vi "Main.vi"() -> ()   [LabVIEW 2017]
uses:
  type defs/action buttons.ctl
  type defs/mode buttons.ctl
  <vilib>/vision/Pattern Matching.llb/IMAQ GM Match Report.ctl
  type defs/data.ctl
  <vilib>/vision/Image Controls.llb/IMAQ Image.ctl
  type defs/states.ctl
  <vilib>/myRIO/Instrument Drivers/Onboard IO/PWM/typedefs/PWM Reference.ctl
  <vilib>/myRIO/Common/Instrument Driver Framework/Utilities/typedefs/myRIO Generic Hardware Reference.ctl
  <vilib>/myRIO/Common/Instrument Driver Framework/Utilities/typedefs/Hardware Version Enum.ctl
  <vilib>/myRIO/Common/Instrument Driver Framework/Utilities/typedefs/myRIO v1.0 Reference.ctl
  <vilib>/myRIO/Common/Instrument Driver Framework/Utilities/typedefs/Generic FPGA Reference.ctl
  <vilib>/myRIO/Common/Instrument Driver Framework/myRIO v1.0/PWM/typedefs/PWM Channels Enum.ctl
  <vilib>/myRIO/Instrument Drivers/Onboard IO/PWM/typedefs/PWM Configuration.ctl
  <vilib>/userdefined/High Color/nirio_resource_hc.ctl
  <vilib>/myRIO/Instrument Drivers/Onboard IO/DIO/typedefs/DIO Reference.ctl
  <vilib>/myRIO/Common/Instrument Driver Framework/myRIO v1.0/DIO/typedefs/DIO Channels List.ctl
  <vilib>/myRIO/Common/Instrument Driver Framework/myRIO v1.0/DIO/typedefs/DIO Channels Enum.ctl
  type defs/task.ctl
  <vilib>/myRIO/Common/Instrument Driver Framework/Utilities/vis/Is FPGA Ref Available.vi
  <vilib>/myRIO/Common/Instrument Driver Framework/myRIO v1.0/PWM/vis/myRIO v1.1 Open PWM.vi
  <vilib>/myRIO/Instrument Drivers/Onboard IO/PWM/vis/Set Duty Cycle and Frequency.vi
  <vilib>/myRIO/Common/Instrument Driver Framework/myRIO v1.0/DIO/vis/myRIO v1.1 Open DIO.vi
  <vilib>/myRIO/Instrument Drivers/Onboard IO/DIO/vis/Write.vi
  <vilib>/myRIO/Instrument Drivers/Onboard IO/DIO/vis/Read.vi
  <vilib>/myRIO/Common/Instrument Driver Framework/Utilities/vis/Validate Channels.vi
  <vilib>/myRIO/Common/Instrument Driver Framework/myRIO v1.0/PWM/vis/myRIO v1.0 Reserve PWM.vi
  <vilib>/myRIO/Common/Instrument Driver Framework/myRIO v1.0/DIO/vis/myRIO v1.0 Reserve DIO.vi
  <vilib>/myRIO/Common/Instrument Driver Framework/myRIO v1.0/UART/vis/myRIO v1.0 Close UART.vi
  <vilib>/myRIO/Common/Instrument Driver Framework/myRIO v1.0/PWM/vis/myRIO v1.0 Build MUX Configuration PWM.vi
  <vilib>/myRIO/Common/Instrument Driver Framework/myRIO v1.0/Resource Manager/vis/myRIO v1.0 Reserve Channel List.vi
  <vilib>/myRIO/Common/Instrument Driver Framework/myRIO v1.0/DIO/vis/myRIO v1.0 Build MUX Configuration DIO.vi
  <vilib>/myRIO/Common/Instrument Driver Framework/myRIO v1.0/Resource Manager/vis/myRIO v1.0 Create Configuration List.vi
  <vilib>/myRIO/Common/Instrument Driver Framework/myRIO v1.0/Resource Manager/vis/myRIO v1.0 Reserve Channel.vi
  <vilib>/myRIO/Common/Instrument Driver Framework/myRIO v1.0/Resource Manager/vis/myRIO v1.0 Unreserve Channel.vi
  <vilib>/myRIO/Common/Instrument Driver Framework/myRIO v1.0/Resource Manager/vis/myRIO v1.0 Build Mutex Name.vi
  <vilib>/Utility/VariantDataType/GetNumericInfo.vi
  <vilib>/Utility/error.llb/Error Cluster From Error Code.vi
  <vilib>/myRIO/Common/Instrument Driver Framework/myRIO v1.0/myRIO v1.1 Open.vi
  <vilib>/myRIO/Common/Instrument Driver Framework/Utilities/vis/IO Manager.vi
  <vilib>/myRIO/Common/Instrument Driver Framework/Utilities/vis/Configuration Manager.vi
  <vilib>/myRIO/Common/Instrument Driver Framework/myRIO v1.0/Resource Manager/vis/myRIO v1.0 Configure IO.vi
  <vilib>/myRIO/Common/Instrument Driver Framework/myRIO v1.0/myRIO v1.0 Close.vi
  <vilib>/myRIO/Common/Instrument Driver Framework/myRIO v1.0/PWM/vis/myRIO v1.0 Write PWM.vi
  <vilib>/myRIO/Common/Instrument Driver Framework/myRIO v1.0/DIO/vis/myRIO v1.0 Write DIO.vi
  <vilib>/myRIO/Common/Instrument Driver Framework/myRIO v1.0/DIO/vis/myRIO v1.0 Read DIO.vi
  <vilib>/myRIO/Common/Instrument Driver Framework/Utilities/vis/FPGA Ref Manager.vi
  <vilib>/myRIO/Common/Instrument Driver Framework/myRIO v1.0/myRIO v1.0 Reset FPGA.vi
  <vilib>/myRIO/Common/Instrument Driver Framework/myRIO v1.0/IRQ/vis/myRIO v1.0 IRQ Info FGV.vi
  <vilib>/myRIO/Common/Instrument Driver Framework/myRIO v1.0/IRQ/vis/myRIO v1.0 Timer IRQ Info FGV.vi
  <vilib>/myRIO/Common/Instrument Driver Framework/myRIO v1.0/IRQ/vis/myRIO v1.0 ISR Agent.vi
  <vilib>/myRIO/Express VI/Onboard IO/PWM/PWM Express VI.xnode
  <vilib>/myRIO/Instrument Drivers/Onboard IO/PWM/vis/myRIO PWM Open.xnode
  <vilib>/myRIO/Express VI/Onboard IO/DO/DO Express VI.xnode
  <vilib>/myRIO/Instrument Drivers/Onboard IO/DIO/vis/myRIO DIO Open.xnode
  <vilib>/myRIO/Express VI/Onboard Devices/LED/LED Express VI.xnode
  <vilib>/myRIO/Express VI/Onboard Devices/Button/Button Express VI.xnode
  <vilib>/vision/NI_Vision_Development_Module.lvlib
  <vilib>/myRIO/Instrument Drivers/Onboard IO/DIO/DIO.lvlib
  <vilib>/myRIO/Instrument Drivers/Onboard IO/PWM/PWM.lvlib
  <vilib>/myRIO/Instrument Drivers/Utilities/Utilities.lvlib
panel:
  out "___Test___":i32[](array[numeric])
  out "data":T1={"Shape - t, Color - f"=FALSE, "qsm"={"Webcam image ref"=refnum, "Analyzed image ref"=refnum, "Stop webcam"=FALSE}, " image ref"=refnum, "number img"=0, "ROI Descriptor (Image Mask 1)"={"Global Rectangle"=[109, 72, 345, 284], "Contours"=[{"ID"=enum."External", "Type"=3, "Coordinates"=[109, 72, 345, 284]}]}, "Pattern class"=0, "Color class"=0, "ROI Descriptor COLOR Mask"={"Global Rectangle"=[109, 72, 345, 284], "Contours"=[{"ID"=enum."External", "Type"=3, "Coordinates"=[109, 72, 345, 284]}]}, "___Test___"=[]} {"ROI Descriptor COLOR Mask"."Contours"."Type" items=["No Selection", "Point", "Line", "Rectangle", "Oval", "Polygon", "Freehand Region", "Annulus", "Unused2", "Unused3", "Broken Line", "Freehand Line", "Rotated Rectangle"]; "ROI Descriptor (Image Mask 1)"."Contours"."Type" items=["No Selection", "Point", "Line", "Rectangle", "Oval", "Polygon", "Freehand Region", "Annulus", "Unused2", "Unused3", "Broken Line", "Freehand Line", "Rotated Rectangle"]}
  in  "ROI Descriptor COLOR Mask":T3={"Global Rectangle"=[109, 72, 345, 284], "Contours"=[{"ID"=enum."External", "Type"=3, "Coordinates"=[109, 72, 345, 284]}]} {"Contours"."Type" items=["No Selection", "Point", "Line", "Rectangle", "Oval", "Polygon", "Freehand Region", "Annulus", "Unused2", "Unused3", "Broken Line", "Freehand Line", "Rotated Rectangle"]}
  in  "Ball index":i32
  out "y0 (circle)":i32
  out "x0 (circle)":i32
  out "x1 (circle)":i32
  out "y1 (circle)":i32
  in  "divider (circle)":sgl=1.0
  out "CircleRadius":dbl
  in  "Look at ball":bool
  in  "x = y?":bool
  in  "y":sgl=1.0
  out "Scale":sgl
  out "error out":errorcluster
  in  "Tab Control":enum32{"Motors", "Shape/Color", "Pattern"}(tab)
  in  "Left+":bool
  in  "Left-":bool
  in  "Right+":bool
  in  "Right-":bool
  in  "M+":bool
  in  "M-":bool
  in  "G+":bool
  in  "G-":bool
  in  "M_PWM":dbl=0.5
  in  "L_PWM":dbl=0.5
  in  "R_PWM":dbl=0.5
  in  "M+ (onGrab)":bool
  out "Circles Calibrated (Shape Detection 1)":T4(array[cluster]) {"Position"."Y" format="%.2f"; "Position"."X" format="%.2f"}
  out "Number of Matches (Shape Detection 1)":i32
  out "Color":i32
  in  "Circle Descriptor (Shape Detection 1)":cluster{"Min Radius":dbl, "Max Radius":dbl}={"Min Radius"=16.0, "Max Radius"=500.0}
  in  "Align X - t, Y - f":bool
  in  "grab time (ms)":u32
  out "Class (Particle Classification 1)":string
  out "y0":i32
  out "x0":i32
  out "x1":i32
  out "y1":i32
  out "Number of Matches (Geometric Matching 1)":i32
  out "Calibrated Matches (Geometric Matching 1)":T5[](array[typedef]) {"Correlation Score" format="%.2f"; "Target Template Curve Score" format="%.2f"; "Template Target Curve Score" format="%.2f"; "Bounding Box"."y" format="%.2f"; "Bounding Box"."x" format="%.2f"; "Position"."y" format="%.2f"; "Position"."x" format="%.2f"; "Score" format="%.2f"; "Scale" format="%.2f"; "Angle" format="%.2f"; "Occlusion %" format="%.2f"}
  out "curY":sgl
  out "curX":sgl
  out "Y is in range":bool
  out "X is in range":bool
  in  "defY":dbl=170.0
  in  "Range":dbl=40.0
  in  "defX":dbl=150.0
  in  "mode buttons":T6
  out "image display":T2(plugin-control)
  in  "action buttons":T7
  in  "Stop":bool
  # "Machine\nVision\nApp"
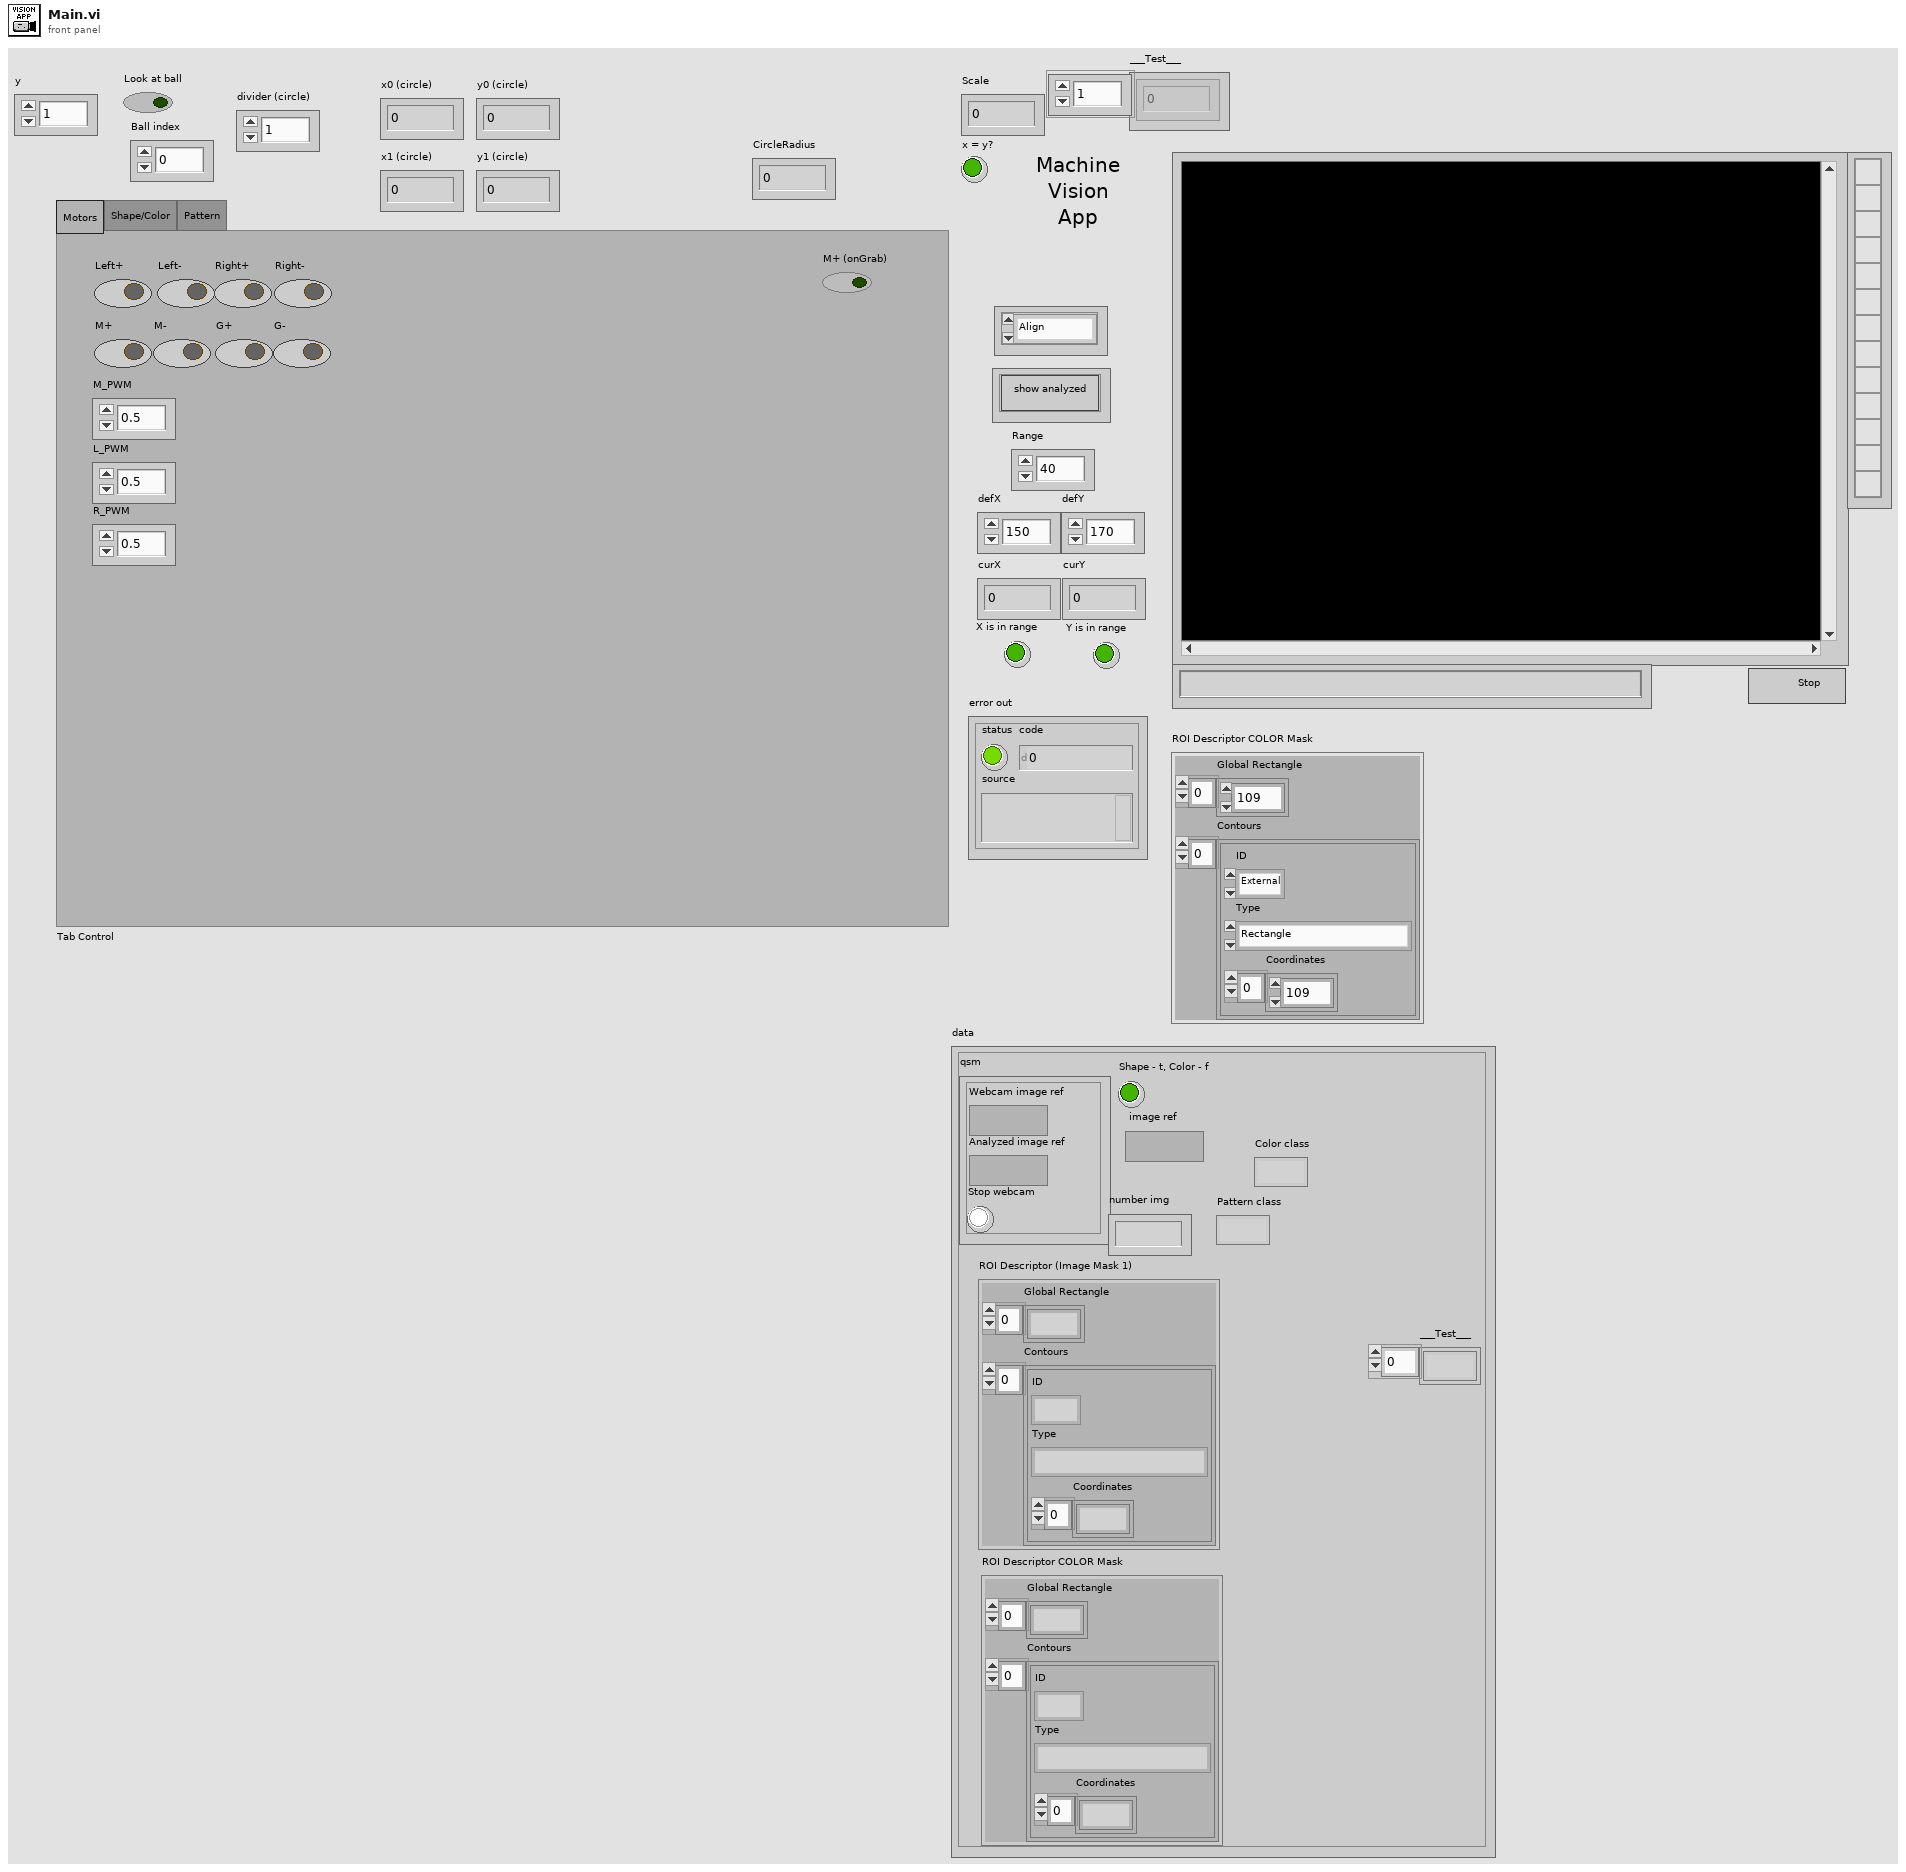
[diagram p1: front panel]
types:
  T1 = typedef "data.ctl" = cluster{"Shape - t, Color - f":bool, "qsm":cluster{"Webcam image ref":T2, "Analyzed image ref":T2, "Stop webcam":bool}, " image ref":T2, "number img":i32, "ROI Descriptor (Image Mask 1)":cluster{"Global Rectangle":i32[], "Contours":cluster{"ID":enum32{"External", "Internal"}, "Type":u32, "Coordinates":i32[]}[]}, "Pattern class":i32, "Color class":i32, "ROI Descriptor COLOR Mask":cluster{"Global Rectangle":i32[], "Contours":cluster{"ID":enum32{"External", "Internal"}, "Type":u32, "Coordinates":i32[]}[]}, "___Test___":i32[]}
  T2 = typedef "IMAQ Image.ctl" = refnum<image>
  T3 = cluster{"Global Rectangle":i32[], "Contours":cluster{"ID":enum32{"External", "Internal"}, "Type":u32, "Coordinates":i32[]}[]}
  T4 = cluster{"Position":cluster{"X":sgl, "Y":sgl}, "Radius":dbl, "Score":dbl}[]
  T5 = typedef "IMAQ GM Match Report.ctl" = cluster{"Position":cluster{"x":sgl, "y":sgl}, "Angle":sgl, "Scale":sgl, "Score":sgl, "Bounding Box":cluster{"x":sgl, "y":sgl}[], "Contrast Reversed":bool, "Occlusion %":sgl, "Template Target Curve Score":sgl, "Target Template Curve Score":sgl, "Correlation Score":sgl}
  T6 = typedef "mode buttons.ctl" = cluster{"show analyzed":bool}
  T7 = typedef "action buttons.ctl" = cluster{"Shape - t, Color - f":enum16{"Align", "Pattern", "Ball", "Other", "Clear", "Joystick control"}}
  T8 = typedef "states.ctl" = enum16{"(qsm) schedule", "(qsm) initialize", "(qsm) release", "(qsm) clean up", "(qsm) shutdown", "(myRIO) initialize", "(myRIO) clean up", "(myRIO) update ports", "(image) get", "(image) analyze", "(image) show", "(ball) Shape detection", "(ball) Calc ball indx", "(ball) Calculate ROI", "X align", "Wait", "Grab", "(pattern) Find Square", "(pattern) Calculate ROI", "(pattern) Analyze pattern", "(joystick) Joystick control", "Wait for button"}
  T9 = typedef "DIO.lvlib/DIO Reference.ctl" = cluster{"myRIO Reference":T10, "DIO Channels List":T14}
  T10 = typedef "myRIO Generic Hardware Reference.ctl" = cluster{"myRIO Model":T11, "myRIO Hardware Reference":T12}
  T11 = typedef "Hardware Version Enum.ctl" = enum16{"Unknown", "myRIO-1900", "myRIO-1950", "roboRIO", "NI ELVIS RIO CM"}
  T12 = typedef "myRIO v1.0 Reference.ctl" = cluster{"Generic FPGA Reference":T13, "Allow multiple opens":bool}
  T13 = typedef "Generic FPGA Reference.ctl" = refnum<k20>
  T14 = typedef "DIO Channels List.ctl" = T15[]
  T15 = typedef "DIO Channels Enum.ctl" = enum16{"Not Connected", "C/DIO0", "C/DIO1", "C/DIO2", "C/DIO3", "C/DIO4", "C/DIO5", "C/DIO6", "C/DIO7", "A/DIO0", "A/DIO1", "A/DIO2", "A/DIO3", "A/DIO4", "A/DIO5", "A/DIO6", "A/DIO7", "A/DIO8", "A/DIO9", "A/DIO10", "A/DIO11", "A/DIO12", "A/DIO13", "A/DIO14", "A/DIO15", "B/DIO0", "B/DIO1", "B/DIO2", "B/DIO3", "B/DIO4", "B/DIO5", "B/DIO6", "B/DIO7", "B/DIO8", "B/DIO9", "B/DIO10", "B/DIO11", "B/DIO12", "B/DIO13", "B/DIO14", "B/DIO15", "LED0", "LED1", "LED2", "LED3", "Button0", "DIO/DIO0", "DIO/DIO1", "DIO/DIO2", "DIO/DIO3", "DIO/DIO4", "DIO/DIO5", "DIO/DIO6", "DIO/DIO7", "DIO/DIO8", "DIO/DIO9", "SPI/CS0", "SPI/CS1", "SPI/CS2", "SPI/CS3", "LED RADIO (Green)", "LED RADIO (Red)", "LED COMM (Green)", "LED COMM (Red)", "LED MODE (Green)", "LED MODE (Red)"}
  T16 = typedef "nirio_resource_hc.ctl" = tag
  T17 = typedef "PWM.lvlib/PWM Reference.ctl" = cluster{"myRIO Reference":T10, "PWM Channels Enum":T18, "PWM Configuration":T19}
  T18 = typedef "PWM Channels Enum.ctl" = enum16{"Not Connected", "C/PWM0", "C/PWM1", "A/PWM0", "A/PWM1", "A/PWM2", "B/PWM0", "B/PWM1", "B/PWM2", "PWM/PWM0", "PWM/PWM1", "PWM/PWM2", "PWM/PWM3", "PWM/PWM4", "PWM/PWM5", "PWM/PWM6", "PWM/PWM7", "PWM/PWM8", "PWM/PWM9"}
  T19 = typedef "PWM.lvlib/PWM Configuration.ctl" = cluster{"Frequency":dbl, "Duty Cycle":dbl}
  T20 = enum16{"Align", "Pattern", "Ball", "Other", "Clear", "Joystick control"}
  T21 = typedef "task.ctl" = T8[]
  T22 = typedef "Image Type" = u32
  T23 = cluster{"Position":cluster{"X":sgl, "Y":sgl}, "Radius":dbl, "Score":dbl}
  T24 = cluster{"ID":enum32{"External", "Internal"}, "Type":u32, "Coordinates":i32[]}[]
  T25 = cluster{"ID":enum32{"External", "Internal"}, "Type":u32, "Coordinates":i32[]}
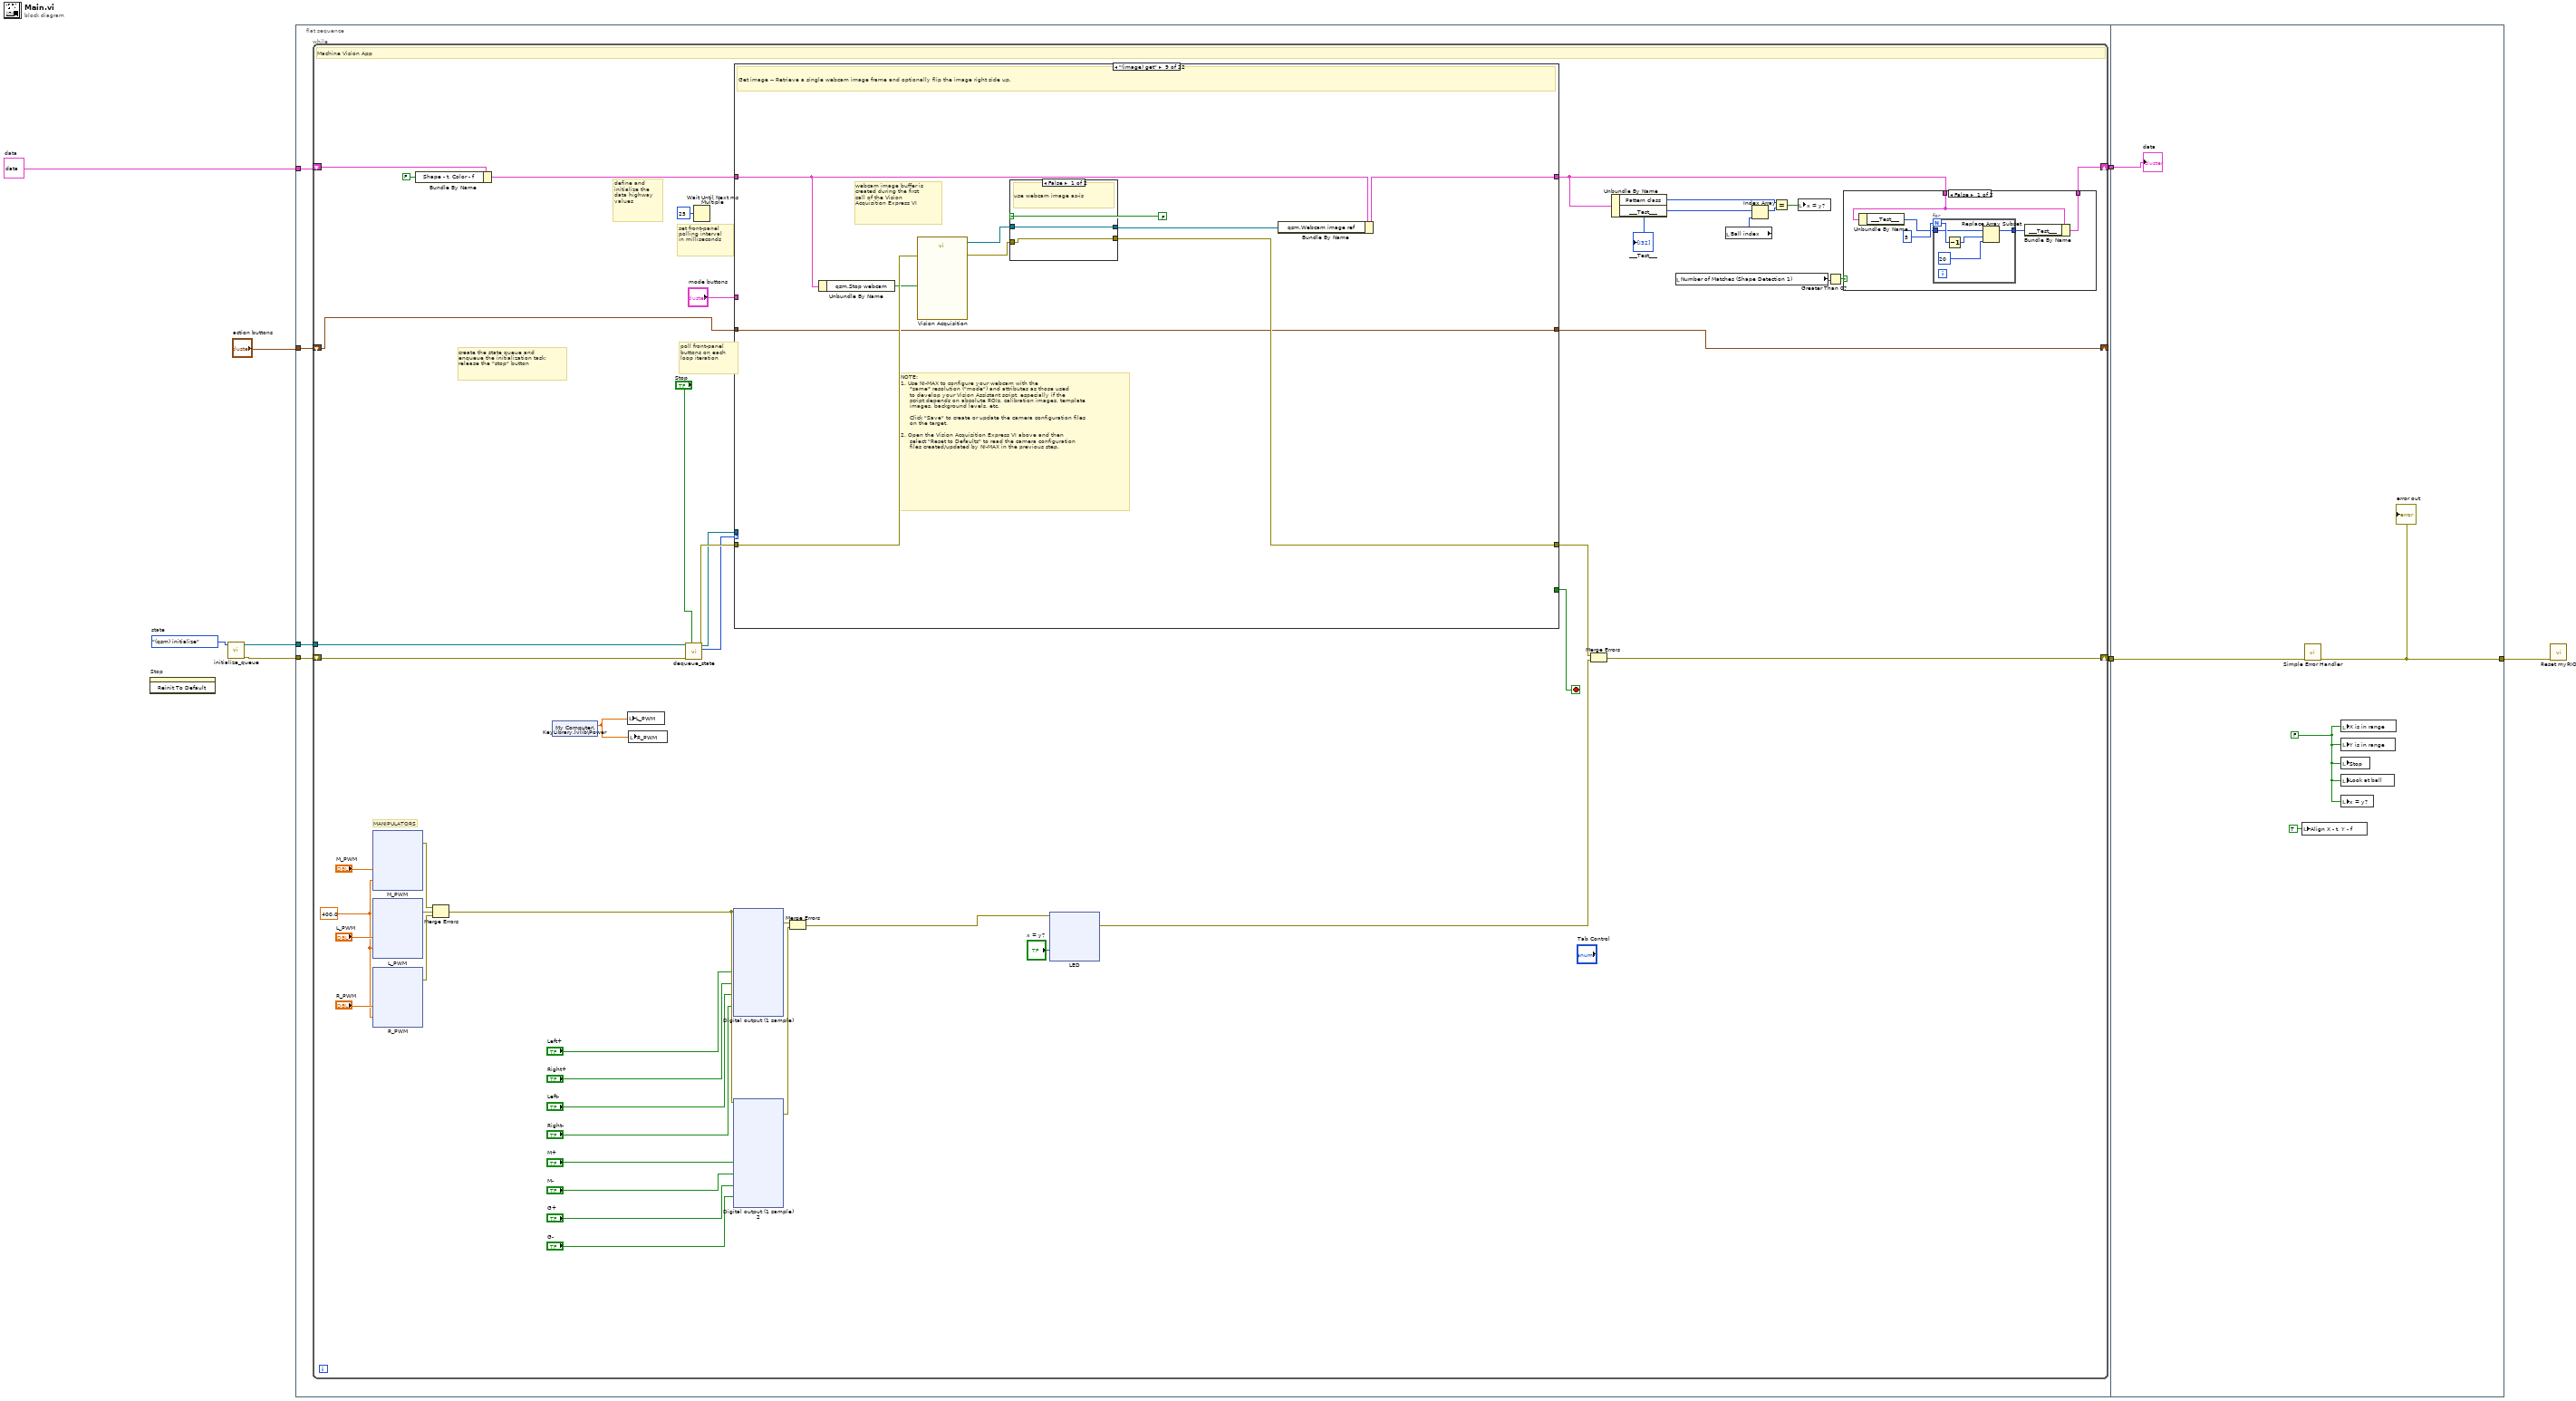
[diagram p0: block diagram]
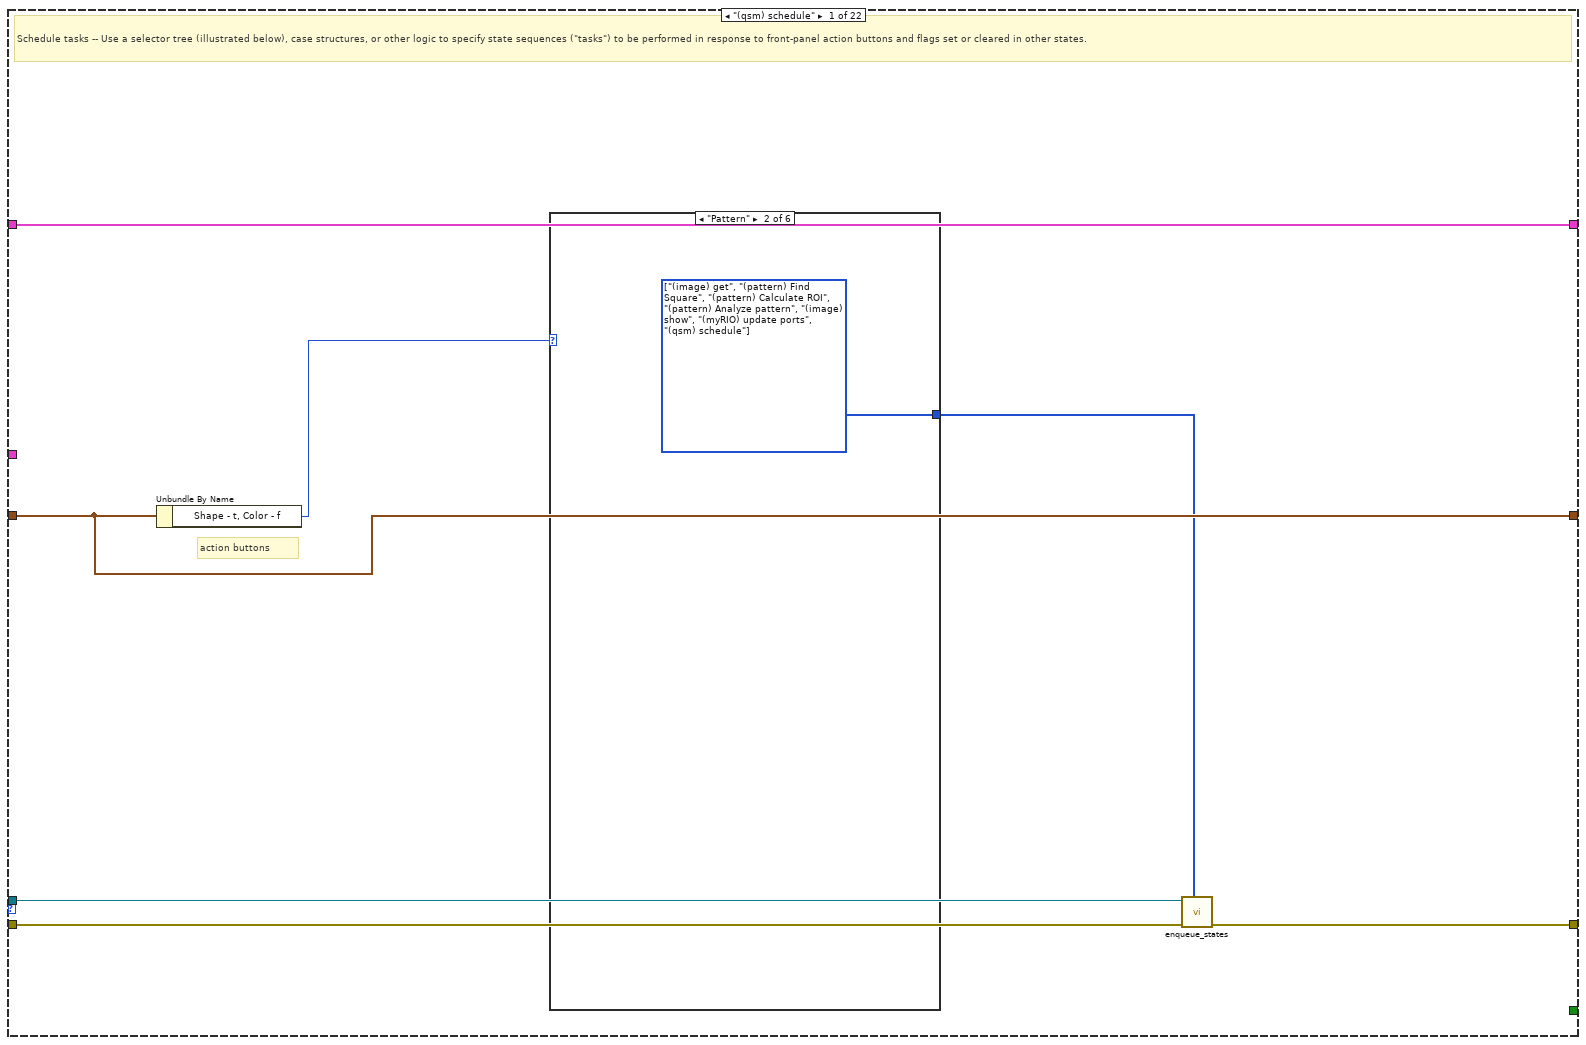
[diagram p3: hidden frame]
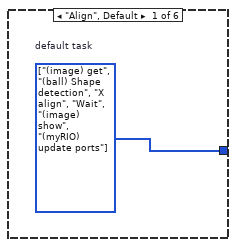
[diagram p4: hidden frame]
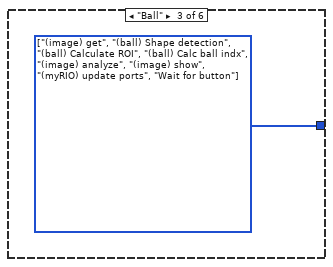
[diagram p5: hidden frame]
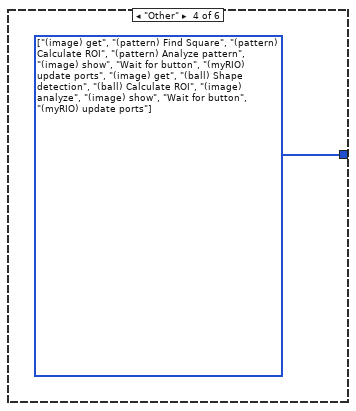
[diagram p6: hidden frame]
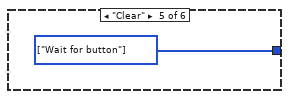
[diagram p7: hidden frame]
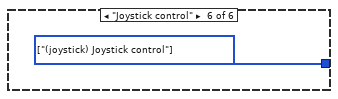
[diagram p8: hidden frame]
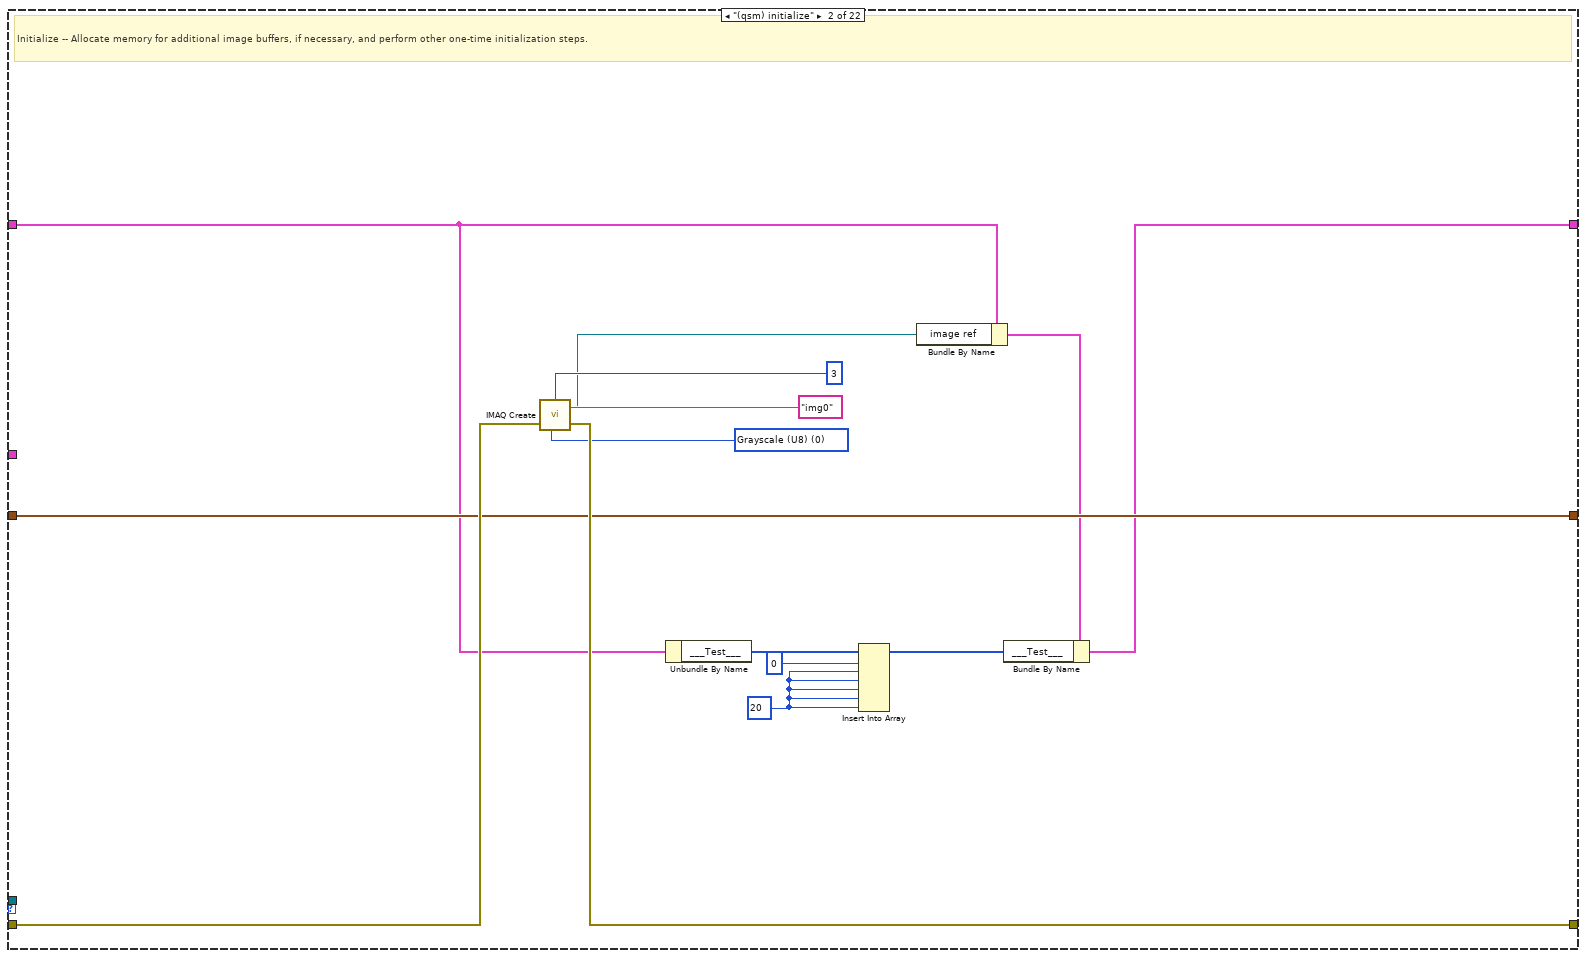
[diagram p9: hidden frame]
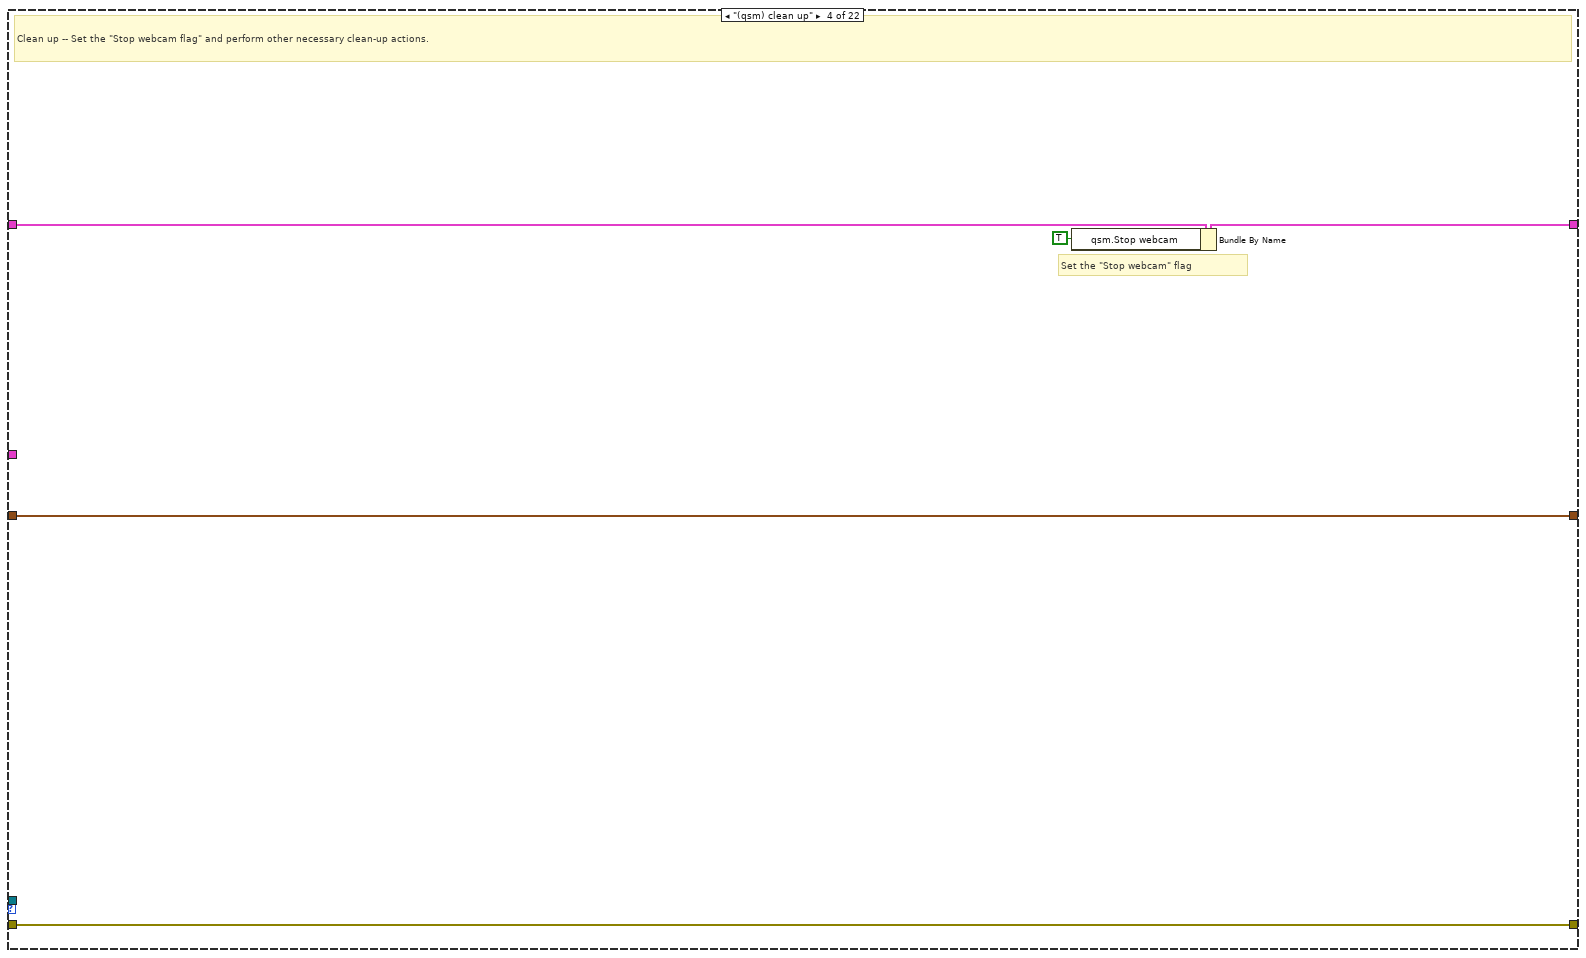
[diagram p11: hidden frame]
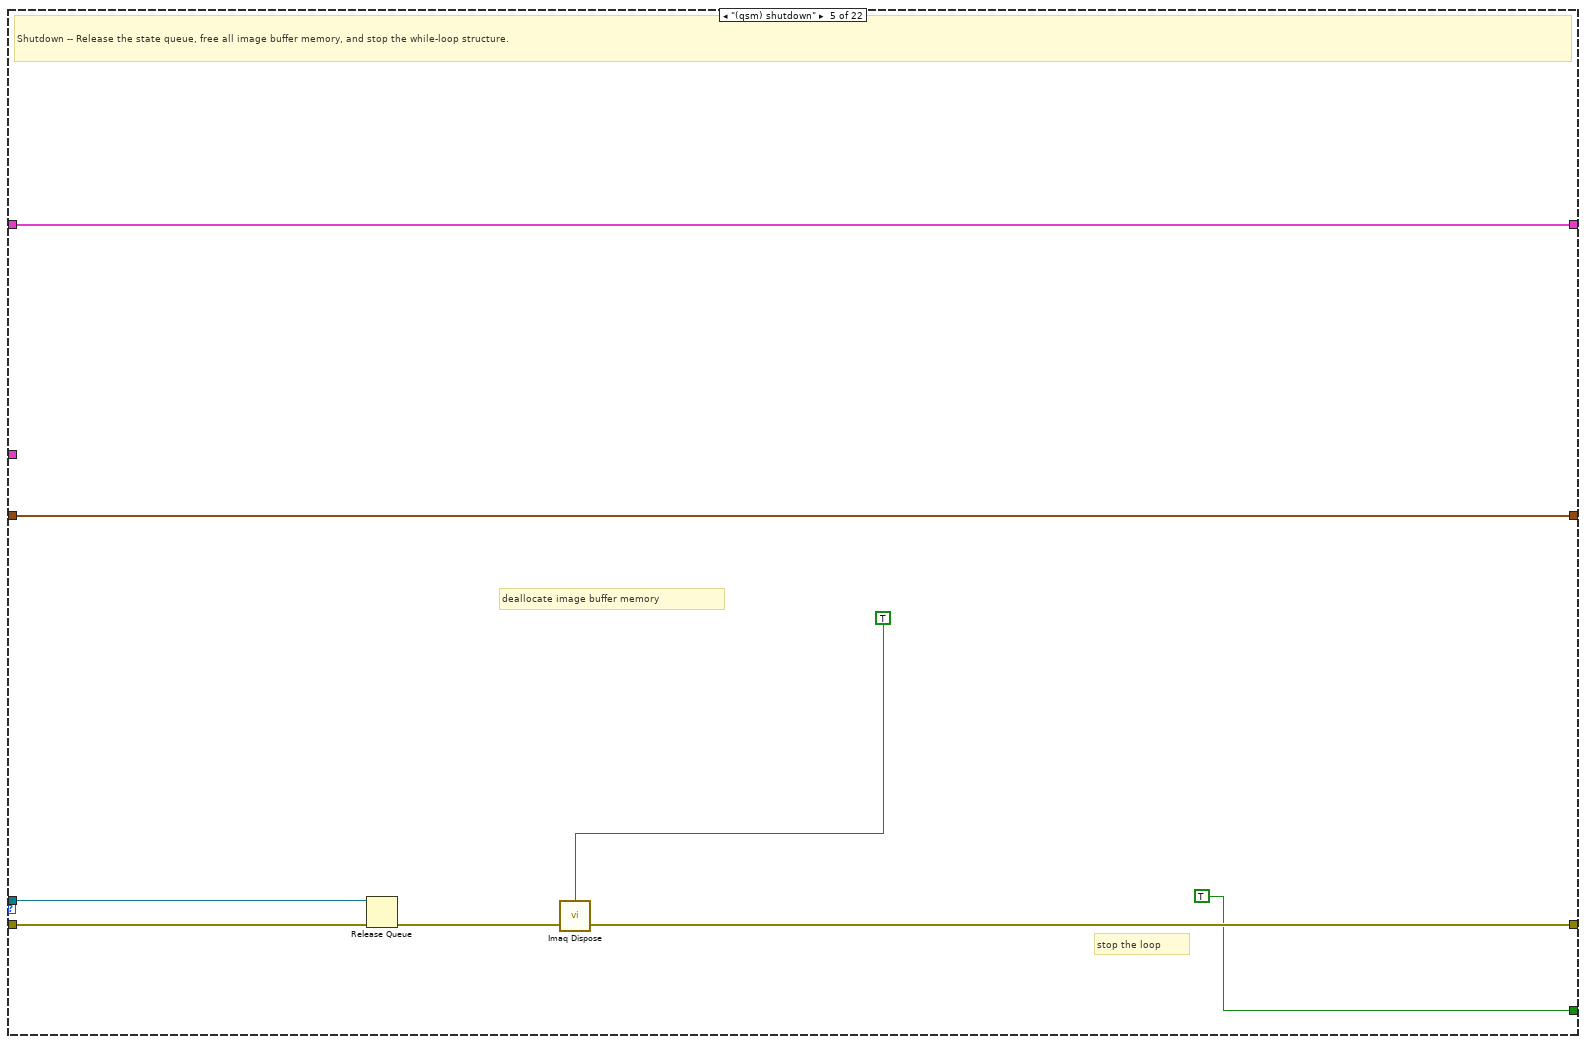
[diagram p12: hidden frame]
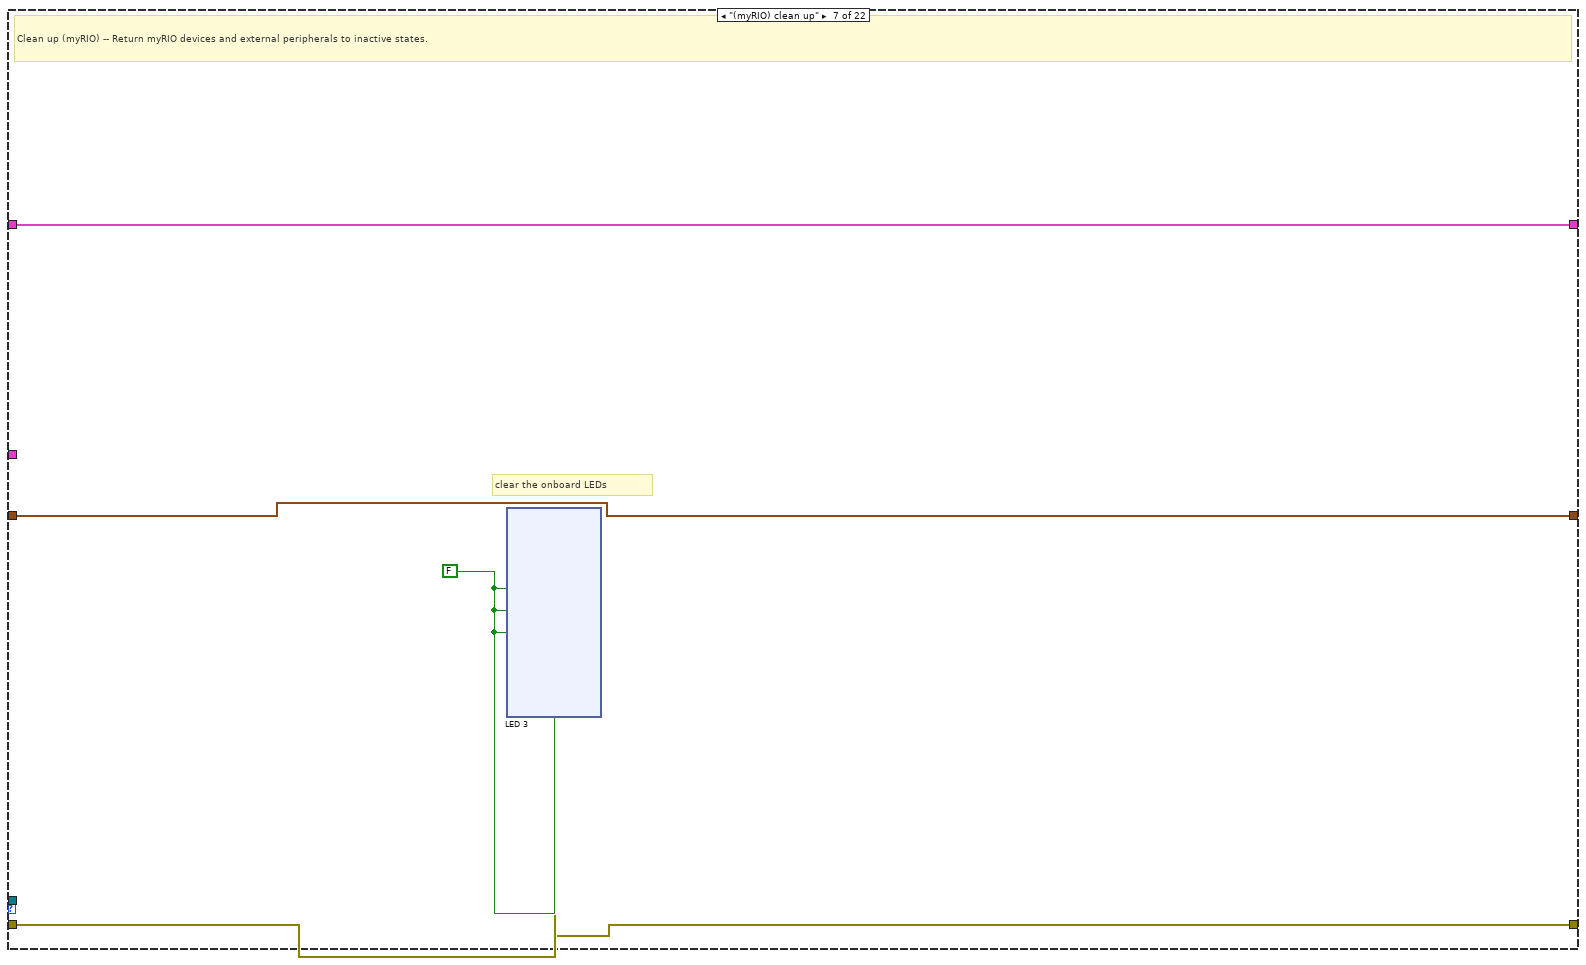
[diagram p14: hidden frame]
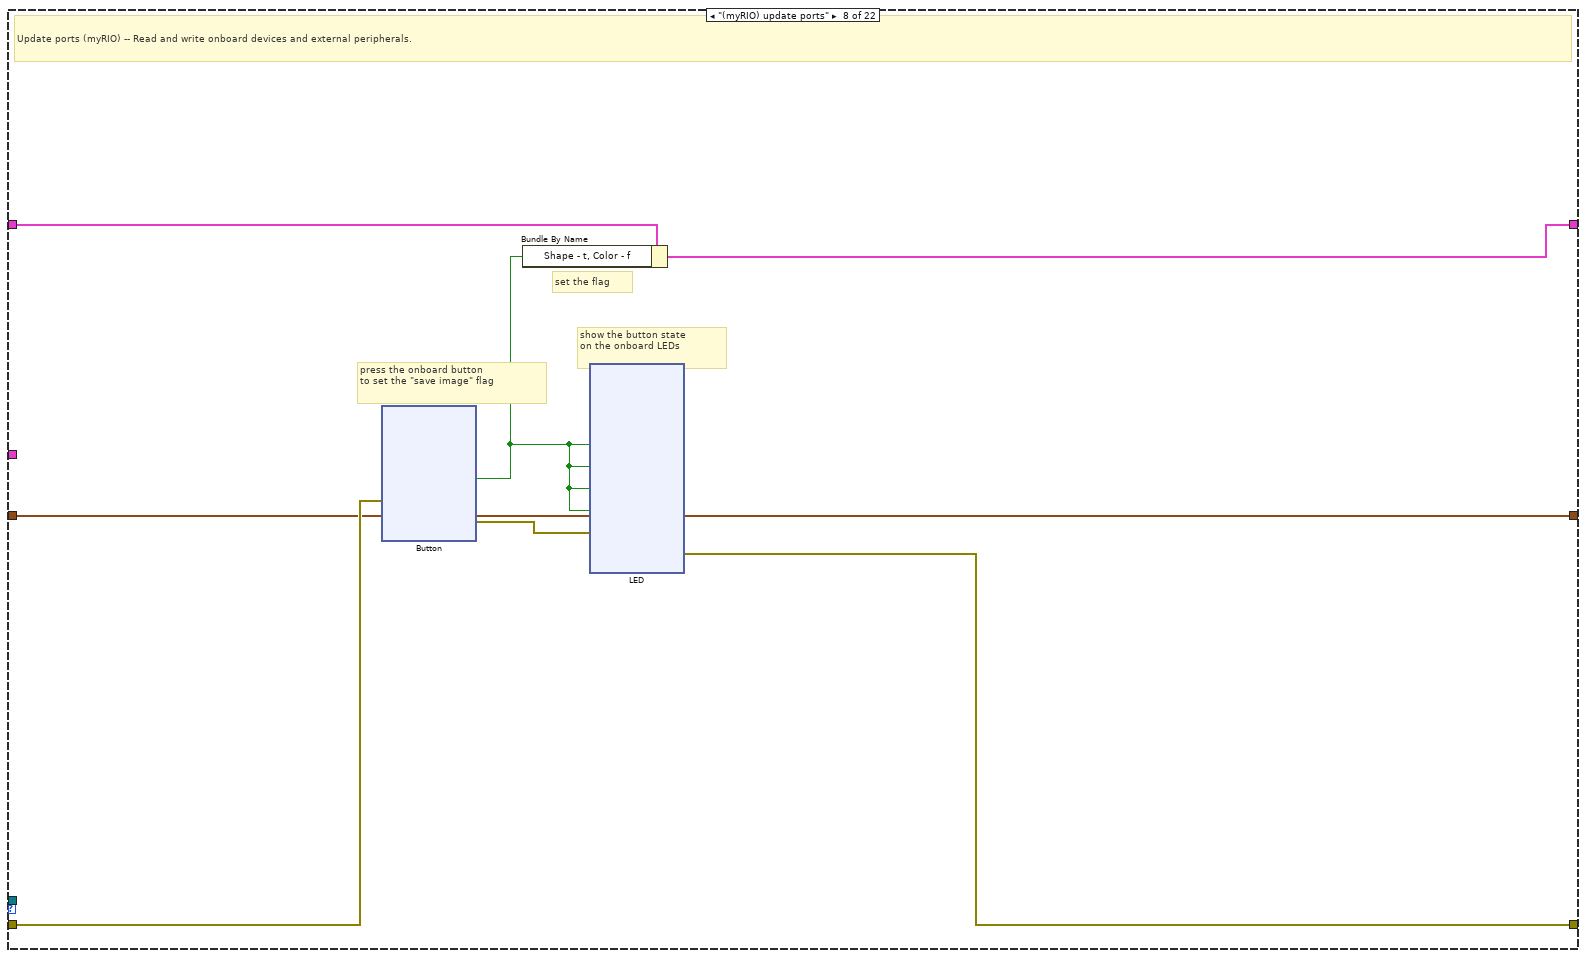
[diagram p15: hidden frame]
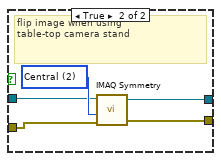
[diagram p16: hidden frame]
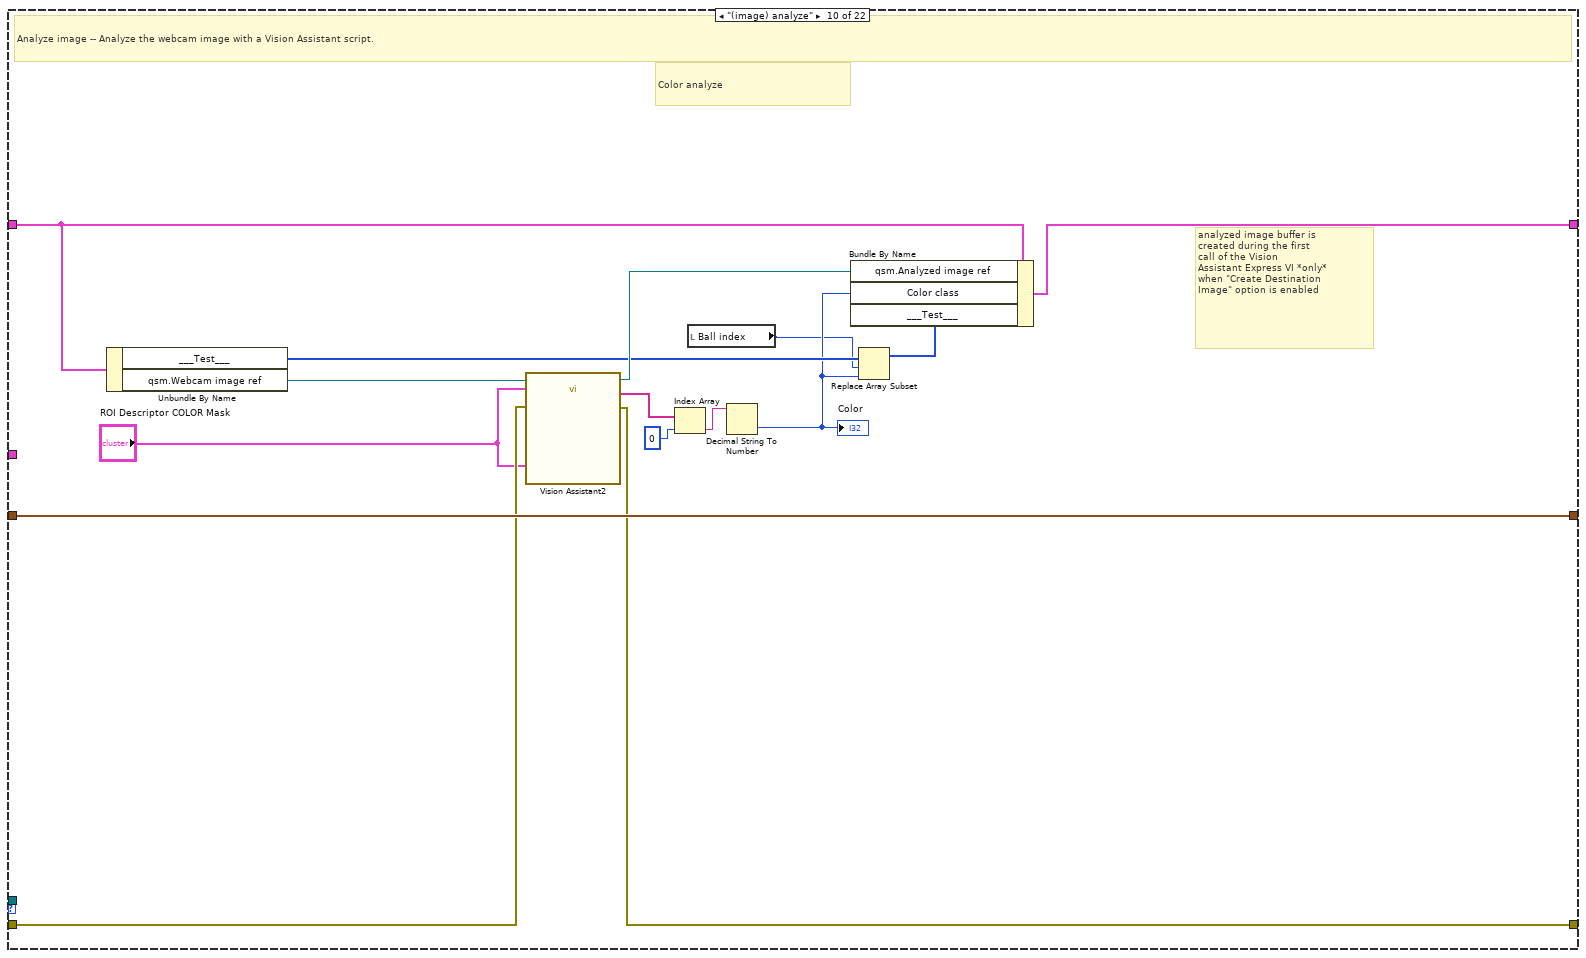
[diagram p17: hidden frame]
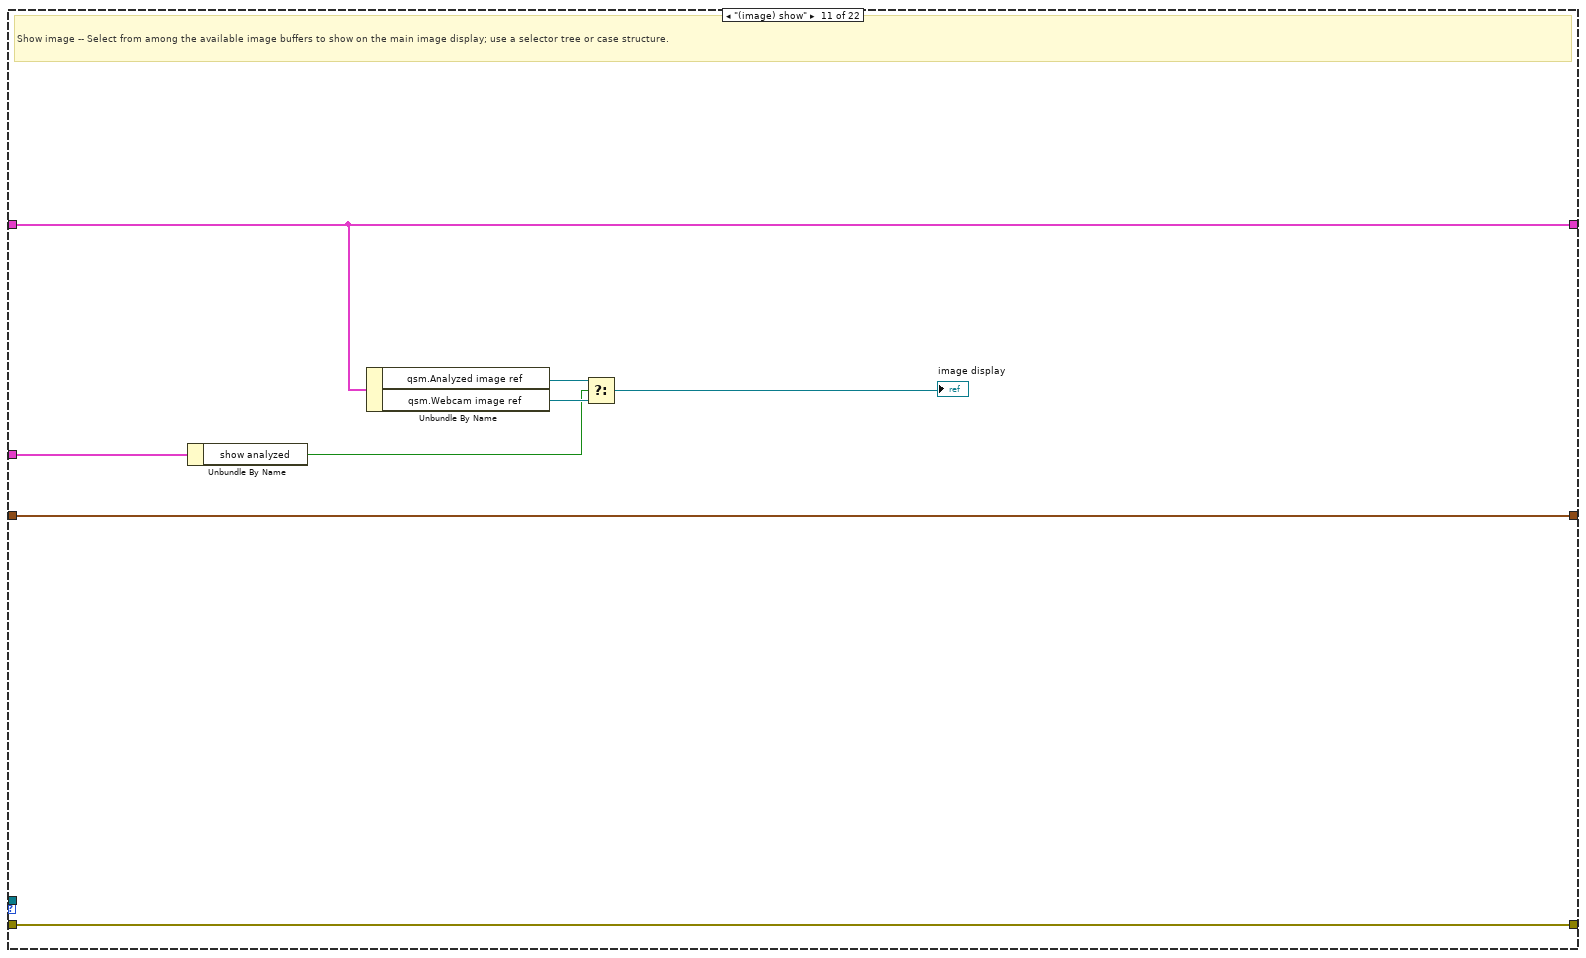
[diagram p18: hidden frame]
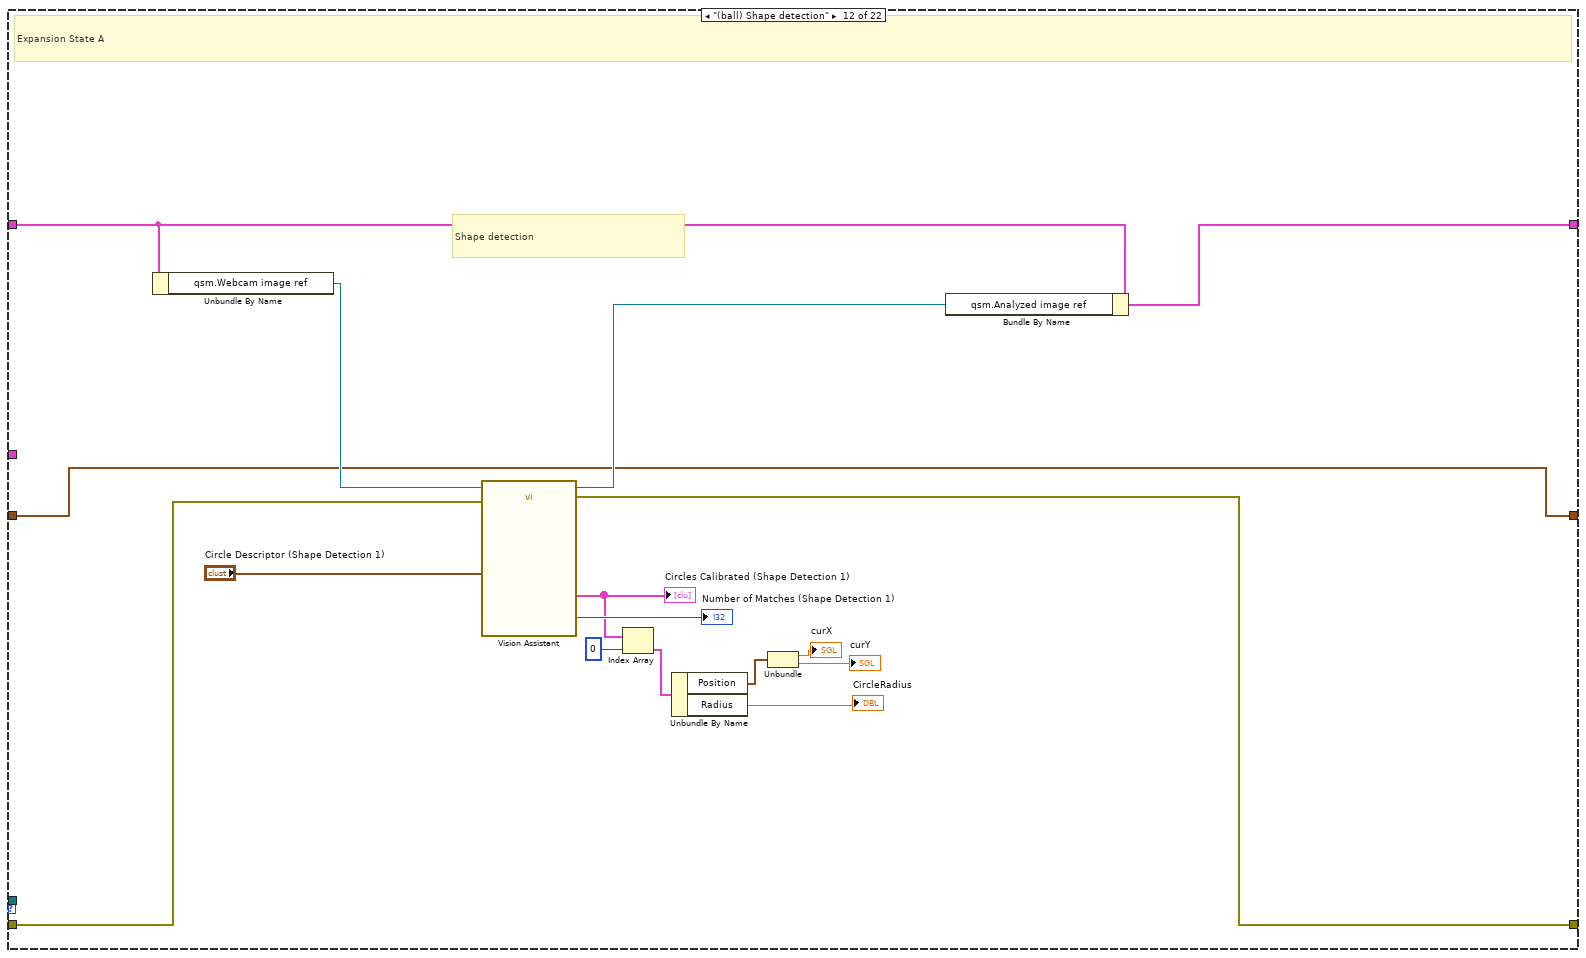
[diagram p19: hidden frame]
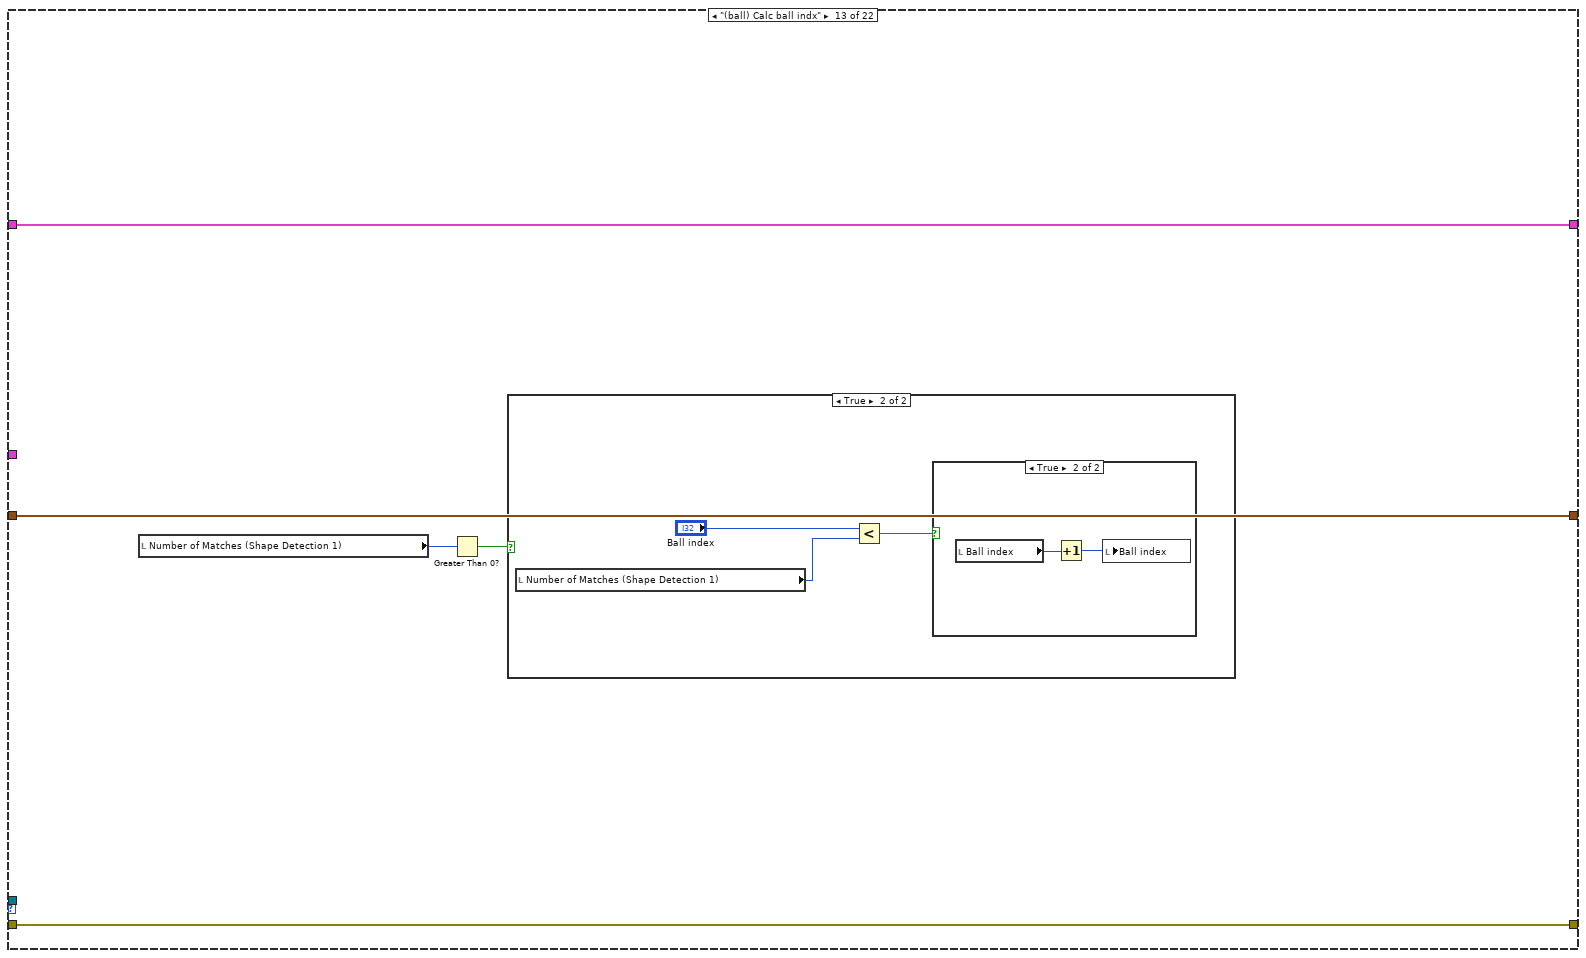
[diagram p20: hidden frame]
diagram:
  w2 = T1 {"Shape - t, Color - f"=FALSE, "qsm"={"Webcam image ref"=refnum, "Analyzed image ref"=refnum, "Stop webcam"=FALSE}, " image ref"=refnum, "number img"=0, "ROI Descriptor (Image Mask 1)"={"Global Rectangle"=[109, 72, 345, 284], "Contours"=[{"ID"=enum."External", "Type"=3, "Coordinates"=[109, 72, 345, 284]}]}, "Pattern class"=0, "Color class"=0, "ROI Descriptor COLOR Mask"={"Global Rectangle"=[51, 157, 345, 350], "Contours"=[{"ID"=enum."External", "Type"=5, "Coordinates"=[137, 230, 93, 226, 75, 199, 49, 200, 56, 145, 98, 111, 200, 119, 250, 126, 235, 166, 240, 212, 188, 243, 303, 244, 336, 247, 336, 271, 335, 292, 335, 318, 314, 323, 293, 334, 279, 345, 272, 349, 187, 349, 186, 335, 120, 334, 112, 314, 100, 297, 59, 291, 51, 288, 51, 287]}]}, "___Test___"=[]}  # data
  w3 = states."(qsm) initialize"  # state
  n1 = invoke on="Stop" class="Bool (strict)" method="Reinit To Default"() -> ()  [unwired: 3 in, 3 out]
  n2 = call "initialize_queue.vi"("state"=w3) -> ("error out"=w4:errorcluster, "queue out"=w5:refnum<queue>)  [unwired: 9 in]
  n3 = flat-sequence {
    tunnel: [w14] -> w7
    tunnel: "action buttons" -> [w13]
    tunnel: w4 -> [w11]
    tunnel: w5 -> [w12]
    tunnel: w2 -> [w10]
    tunnel: [w9] -> w1
    tunnel: [w866] -> w8
    tunnel: w7 -> [w867]
    tunnel: w1 -> [w865]
    frame #0 {
      n4 = while {
        shift-right: [w55] -> w14
        shift-left: w11 -> [w60]
        shift-right: [w22] -> w9
        shift-left: w10 -> [w36]
        shift-right: [w35] -> _
        shift-left: w13 -> [w34]
        tunnel: w12 -> [w33]
        stop <- w31 stop-if-true
        w38 = 400.0 ("Frequency [Hz]")
        # "define and \ninitialize the \ndata highway\nvalues"
        # "MANIPULATORS"
        # "create the state queue and\nenqueue the initialization task;\nrelease the \"stop\" button"
        # "set front-panel\npolling interval\nin milliseconds"
        # "poll front-panel\nbuttons on each\nloop iteration"
        # "Machine Vision App"
        n5 = xnode "M_PWM"("Duty Cycle"="M_PWM", "Frequency [Hz]"=w38) -> ("error out"=w54:errorcluster)  [unwired: 1 in]
        n6 = xnode "L_PWM"("Duty Cycle"="L_PWM", "Frequency [Hz]"=w38) -> ("error out"=w53:errorcluster)  [unwired: 1 in]
        n7 = xnode "R_PWM"("Duty Cycle"="R_PWM", "Frequency [Hz]"=w38) -> ("error out"=w52:errorcluster)  [unwired: 1 in]
        n8 = Bundle By Name(cluster=w36, "Shape - t, Color - f"=FALSE) -> (w30:T1)
        n9 = Merge Errors(w54, w53, w52) -> (w49:errorcluster)
        n10 = shared-variable "My Computer\\KeyLibrary.lvlib\\Power"() -> (w15:dbl)  [unwired: 1 in, 1 out]
        n11 = local write "L_PWM"(w15) -> ()
        n12 = local write "R_PWM"(w15) -> ()
        n13 = call "dequeue_state.vi"("stop"="Stop", "error in (no error)"=w60, "queue in"=w33) -> ("error out"=w61:errorcluster, "state"=w56:T8, "queue out"=w37:refnum<queue>)  [unwired: 6 in]
        n14 = Wait Until Next ms Multiple(millisecond multiple=u32 25) -> ()  [unwired: 1 out]
        n15 = xnode "Digital output (1 sample)"("Left+ (A/DIO5 (Pin 21))"="Left+", "Right+ (A/DIO7 (Pin 25))"="Right+", "Left- (A/DIO6 (Pin 23))"="Left-", "Right- (A/DIO13 (Pin 26))"="Right-", "error in (no error)"=w49) -> ("error out"=w51:errorcluster)
        n16 = xnode "Digital output (1 sample) 2"("M+ (B/DIO5 (Pin 21))"="M+", "M- (B/DIO6 (Pin 23))"="M-", "G+ (B/DIO7 (Pin 25))"="G+", "G- (B/DIO13 (Pin 26))"="G-", "error in (no error)"=w49) -> ("error out"=w50:errorcluster)
        n17 = case shown="\"(image) get\"" w56 {
          tunnel: w61 -> [w292 w315 w317 w320 w331 w333 w337 w382 w462 w481 w493 w513 w515 w525 w575 w611 w630 w710 w723 w772 w789 w860]
          tunnel: w37 -> [w293 _ _ _ w330 _ _ _ _ _ _ _ _ _ w574 w609 _ _ _ _ _ _]
          tunnel: [w294 w314 w317 w320 w326 w333 w336 w380 w465 w482 w493 w508 w515 w525 w575 w610 w629 w711 w723 w773 w788 w860] -> w19
          tunnel: w34 -> [w291 w309 w316 w319 w325 w332 w335 w378 w458 w486 w490 w504 w514 w524 w572 w613 w631 w718 w720 w776 w807 w861]
          tunnel: w30 -> [w295 w306 w318 w322 w329 w334 w339 w384 w463 w489 w494 w510 w516 w527 w576 w615 w632 w714 w721 w779 w808 w858]
          tunnel: [w295 w307 w318 w321 w329 w334 w339 w383 w467 w488 w494 w509 w516 w526 w576 w614 w632 w713 w722 w778 w808 w858] -> w23
          tunnel: "mode buttons" -> [_ _ _ _ _ _ _ _ _ _ w492 _ _ _ _ _ _ _ _ _ _ _]
          tunnel: [w291 w309 w316 w319 w325 w332 w335 w378 w458 w486 w490 w504 w514 w524 w572 w612 w631 w718 w720 w776 w807 w861] -> w35
          tunnel: [_ _ _ _ TRUE _ _ _ _ _ _ _ _ _ _ _ _ _ _ _ _ _] -> w31
          frame "(qsm) schedule" {
            # "action buttons"
            # "Schedule tasks -- Use a selector tree (illustrated below), case structures, or other logic to specify state sequences (\"tasks\") to be performed in response to front-panel action buttons and flags set or cleared in other states."
            n18 = Unbundle By Name(w291) -> ("Shape - t, Color - f"=w290:T20)
            n19 = case shown="\"Pattern\"" w290 {
              tunnel: [w296 w297 w298 w299 w300 w301] -> w289
              frame "Align", Default {
                w296 = T21 [enum."(image) get", enum."(ball) Shape detection", enum."X align", enum."Wait", enum."(image) show", enum."(myRIO) update ports"] items=["(qsm) schedule", "(qsm) initialize", "(qsm) release", "(qsm) clean up", "(qsm) shutdown", "(myRIO) initialize", "(myRIO) clean up", "(myRIO) update ports", "(image) get", "(image) analyze", "(image) show", "(ball) Shape detection", "(ball) Calc ball indx", "(ball) Calculate ROI", "X align", "Wait", "Grab", "(pattern) Find Square", "(pattern) Calculate ROI", "(pattern) Analyze pattern", "(joystick) Joystick control", "Wait for button"]  # default task
              }
              frame "Pattern" {
                w297 = T21 [enum."(image) get", enum."(pattern) Find Square", enum."(pattern) Calculate ROI", enum."(pattern) Analyze pattern", enum."(image) show", enum."(myRIO) update ports", enum."(qsm) schedule"] items=["(qsm) schedule", "(qsm) initialize", "(qsm) release", "(qsm) clean up", "(qsm) shutdown", "(myRIO) initialize", "(myRIO) clean up", "(myRIO) update ports", "(image) get", "(image) analyze", "(image) show", "(ball) Shape detection", "(ball) Calc ball indx", "(ball) Calculate ROI", "X align", "Wait", "Grab", "(pattern) Find Square", "(pattern) Calculate ROI", "(pattern) Analyze pattern", "(joystick) Joystick control", "Wait for button"] ("task")
              }
              frame "Ball" {
                w298 = T21 [enum."(image) get", enum."(ball) Shape detection", enum."(ball) Calculate ROI", enum."(ball) Calc ball indx", enum."(image) analyze", enum."(image) show", enum."(myRIO) update ports", enum."Wait for button"] items=["(qsm) schedule", "(qsm) initialize", "(qsm) release", "(qsm) clean up", "(qsm) shutdown", "(myRIO) initialize", "(myRIO) clean up", "(myRIO) update ports", "(image) get", "(image) analyze", "(image) show", "(ball) Shape detection", "(ball) Calc ball indx", "(ball) Calculate ROI", "X align", "Wait", "Grab", "(pattern) Find Square", "(pattern) Calculate ROI", "(pattern) Analyze pattern", "(joystick) Joystick control", "Wait for button"] ("task")
              }
              frame "Other" {
                w299 = T21 [enum."(image) get", enum."(pattern) Find Square", enum."(pattern) Calculate ROI", enum."(pattern) Analyze pattern", enum."(image) show", enum."Wait for button", enum."(myRIO) update ports", enum."(image) get", enum."(ball) Shape detection", enum."(ball) Calculate ROI", enum."(image) analyze", enum."(image) show", enum."Wait for button", enum."(myRIO) update ports"] items=["(qsm) schedule", "(qsm) initialize", "(qsm) release", "(qsm) clean up", "(qsm) shutdown", "(myRIO) initialize", "(myRIO) clean up", "(myRIO) update ports", "(image) get", "(image) analyze", "(image) show", "(ball) Shape detection", "(ball) Calc ball indx", "(ball) Calculate ROI", "X align", "Wait", "Grab", "(pattern) Find Square", "(pattern) Calculate ROI", "(pattern) Analyze pattern", "(joystick) Joystick control", "Wait for button"] ("task")
              }
              frame "Clear" {
                w300 = T21 [enum."Wait for button"] items=["(qsm) schedule", "(qsm) initialize", "(qsm) release", "(qsm) clean up", "(qsm) shutdown", "(myRIO) initialize", "(myRIO) clean up", "(myRIO) update ports", "(image) get", "(image) analyze", "(image) show", "(ball) Shape detection", "(ball) Calc ball indx", "(ball) Calculate ROI", "X align", "Wait", "Grab", "(pattern) Find Square", "(pattern) Calculate ROI", "(pattern) Analyze pattern", "(joystick) Joystick control", "Wait for button"]
              }
              frame "Joystick control" {
                w301 = T21 [enum."(joystick) Joystick control"] items=["(qsm) schedule", "(qsm) initialize", "(qsm) release", "(qsm) clean up", "(qsm) shutdown", "(myRIO) initialize", "(myRIO) clean up", "(myRIO) update ports", "(image) get", "(image) analyze", "(image) show", "(ball) Shape detection", "(ball) Calc ball indx", "(ball) Calculate ROI", "X align", "Wait", "Grab", "(pattern) Find Square", "(pattern) Calculate ROI", "(pattern) Analyze pattern", "(joystick) Joystick control", "Wait for button"]
              }
            }
            n20 = call "enqueue_states.vi"("task"=w289, "error in"=w292, "queue in"=w293) -> ("error out"=w294:errorcluster)  [unwired: 6 in, 1 out]
          }
          frame "(qsm) initialize" {
            w302 = 20
            w312 = T22 0 items=["Grayscale (U8)", "Grayscale (I16)", "Grayscale (SGL)", "Complex (CSG)", "RGB (U32)", "HSL (U32)", "RGB (U64)", "Grayscale (U16)"] ("Image Type")
            # "Initialize -- Allocate memory for additional image buffers, if necessary, and perform other one-time initialization steps."
            n21 = call "IMAQ Create"("Border Size"=3, "Image Name"="img0", "Image Type"=w312, "error in (no error)"=w315) -> ("New Image"=w310:T2, "error out"=w314:errorcluster)  [unwired: 1 in]
            n22 = Unbundle By Name(w306) -> ("___Test___"=w303:i32[])
            n23 = Insert Into Array(array=w303, index=0, new element #1=w302, new element #2=w302, new element #3=w302, new element #4=w302, new element #5=w302) -> (w305:i32[])
            n24 = Bundle By Name(cluster=w306, "image ref"=w310) -> (w308:T1)
            n25 = Bundle By Name(cluster=w308, "___Test___"=w305) -> (w307:T1)
          }
          frame "(qsm) release" {
            # "Release all front-panel action buttons."
          }
          frame "(qsm) clean up" {
            # "Set the \"Stop webcam\" flag"
            # "Clean up -- Set the \"Stop webcam flag\" and perform other necessary clean-up actions."
            n26 = Bundle By Name(cluster=w322, "qsm.Stop webcam"=TRUE) -> (w321:T1)
          }
          frame "(qsm) shutdown" {
            # "deallocate image buffer memory"
            # "stop the loop"
            # "Shutdown -- Release the state queue, free all image buffer memory, and stop the while-loop structure."
            n27 = Release Queue(queue=w330, error in (no error)=w331) -> (error out=w327:errorcluster)  [unwired: 1 in, 2 out]
            n28 = call "Imaq Dispose"("All Images? (No)"=TRUE, "error in (no error)"=w327) -> ("error out"=w326:errorcluster)  [unwired: 4 in]
          }
          frame "(myRIO) initialize" {
            # "Initialize (myRIO) -- Open channels, configure devices, send setup strings to peripherals, etc."
          }
          frame "(myRIO) clean up" {
            w338 = FALSE ("LED3")
            # "clear the onboard LEDs"
            # "Clean up (myRIO) -- Return myRIO devices and external peripherals to inactive states."
            n29 = xnode "LED 3"("LED0"=w338, "LED1"=w338, "LED2"=w338, "LED3"=w338, "error in (no error)"=w337) -> ("error out"=w336:errorcluster)
          }
          frame "(myRIO) update ports" {
            # "show the button state\non the onboard LEDs"
            # "set the flag"
            # "press the onboard button\nto set the \"save image\" flag"
            # "Update ports (myRIO) -- Read and write onboard devices and external peripherals."
            n30 = xnode "Button"("error in (no error)"=w382) -> ("Value"=w379:bool, "error out"=w381:errorcluster)
            n31 = Bundle By Name "Bundle By Name"(cluster=w384, "Shape - t, Color - f"=w379) -> (w383:T1)
            n32 = xnode "LED"("LED0"=w379, "LED1"=w379, "LED2"=w379, "LED3"=w379, "error in (no error)"=w381) -> ("error out"=w380:errorcluster)
          }
          frame "(image) get" {
            # "NOTE:\n1. Use NI-MAX to configure your webcam with the\n     *same* resolution (\"mode\") and attributes as those used \n     to develop your Vision Assistant script, especially if the\n     script depends on absolute ROIs, calibration images, template\n     images, background levels, etc.\n \n     Click \"Save\" to create or update the camera configuration files\n     on the target.\n\n2. Open the Vision Acquisition Express VI above and then\n     select \"Reset to Defaults\" to read the camera configuration\n     files created/updated by NI-MAX in the previous step."
            # "webcam image buffer is\ncreated during the first\ncall of the Vision\nAcquisition Express VI"
            # "Get image -- Retrieve a single webcam image frame and optionally flip the image right side up."
            n33 = Unbundle By Name(w463) -> ("qsm.Stop webcam"=w461:bool)
            n34 = call "Vision Acquisition"("Stop (F)"=w461, "error in"=w462) -> ("Image Out"=w460:T2, "error out"=w459:errorcluster)  [unwired: 22 in, 2 out]
            n35 = case shown="False" FALSE {
              tunnel: w460 -> [w469 w473]
              tunnel: [w469 w472] -> w466
              tunnel: w459 -> [w468 w471]
              tunnel: [w468 w470] -> w465
              frame False {
                # "use webcam image as-is"
              }
              frame True {
                w474 = u32 2 items=["Horizontal", "Vertical", "Central", "1st Diagonal", "2nd Diagonal"] ("Type of Symmetry")
                # "flip image when using\ntable-top camera stand"
                n36 = call "IMAQ Symmetry"("error in (no error)"=w471, "Type of Symmetry"=w474, "Image Src"=w473) -> ("error out"=w470:errorcluster, "Image Dst Out"=w472:T2)  [unwired: 2 in]
              }
            }
            n37 = Bundle By Name(cluster=w463, "qsm.Webcam image ref"=w466) -> (w467:T1)
          }
          frame "(image) analyze" {
            # "Color analyze"
            # "analyzed image buffer is\ncreated during the first\ncall of the Vision\nAssistant Express VI *only*\nwhen \"Create Destination\nImage\" option is enabled"
            # "Analyze image -- Analyze the webcam image with a Vision Assistant script."
            n38 = Unbundle By Name "Unbundle By Name"(w489) -> ("___Test___"=w477:i32[], "qsm.Webcam image ref"=w485:T2)
            n39 = call "Vision Assistant2"("Image In"=w485, "ROI Descriptor (Color Classification 1)"="ROI Descriptor COLOR Mask", "ROI Descriptor (Image Mask 1)"="ROI Descriptor COLOR Mask", "error in"=w481) -> ("Image Out"=w484:T2, "Classes (Color Classification 1)"=w483:string[], "error out"=w482:errorcluster)  [unwired: 21 in]
            n40 = Index Array(array=w483, index=0) -> (element=w487:string)
            n41 = local read "Ball index"() -> (w475:i32)
            n42 = Decimal String To Number(string=w487) -> (number=w476:i32)  [unwired: 2 in, 1 out]
            "Color" <- w476
            n43 = Replace Array Subset(array=w477, new element=w476, index=w475) -> (w478:i32[])
            n44 = Bundle By Name "Bundle By Name"(cluster=w489, "qsm.Analyzed image ref"=w484, "Color class"=w476, "___Test___"=w478) -> (w488:T1)
          }
          frame "(image) show" {
            # "Show image -- Select from among the available image buffers to show on the main image display; use a selector tree or case structure."
            n45 = Unbundle By Name "Unbundle By Name"(w492) -> ("show analyzed"=w491:bool)
            n46 = Unbundle By Name "Unbundle By Name"(w494) -> ("qsm.Analyzed image ref"=w497:T2, "qsm.Webcam image ref"=w496:T2)
            n47 = Select(t=w497, s=w491, f=w496) -> (s? t:f=→"image display":T2)
          }
          frame "(ball) Shape detection" {
            # "Shape detection"
            # "Expansion State A"
            n48 = Unbundle By Name(w510) -> ("qsm.Webcam image ref"=w512:T2)
            n49 = call "Vision Assistant"("Image In"=w512, "error in"=w513, "Circle Descriptor (Shape Detection 1)"="Circle Descriptor (Shape Detection 1)") -> ("Image Out"=w511:T2, "error out"=w508:errorcluster, "Circles Calibrated (Shape Detection 1)"=w506:T4, "Number of Matches (Shape Detection 1)"=→"Number of Matches (Shape Detection 1)":i32)  [unwired: 21 in]
            "Circles Calibrated (Shape Detection 1)" <- w506
            n50 = Index Array(array=w506, index=0) -> (element=w502:T23)
            n51 = Unbundle By Name(w502) -> ("Position"=w501:cluster{"X":sgl, "Y":sgl}, "Radius"=→"CircleRadius":dbl)
            n52 = Unbundle(w501) -> ("X"=→"curX":sgl, "Y"=→"curY":sgl)
            n53 = Bundle By Name(cluster=w510, "qsm.Analyzed image ref"=w511) -> (w509:T1)
          }
          frame "(ball) Calc ball indx" {
            n54 = local read "Number of Matches (Shape Detection 1)"() -> (w518:i32)
            n55 = Greater Than 0?(x=w518) -> (x > 0?=w517:bool)
            n56 = case shown="True" w517 {
              frame False {
              }
              frame True {
                n57 = local read "Number of Matches (Shape Detection 1)"() -> (w520:i32)
                n58 = Less?(x="Ball index", y=w520) -> (x < y?=w519:bool)
                n59 = case shown="True" w519 {
                  frame False {
                  }
                  frame True {
                    n60 = local read "Ball index"() -> (w523:i32)
                    n61 = Increment(x=w523) -> (x+1=w522:i32)
                    n62 = local write "Ball index"(w522) -> ()
                  }
                }
              }
            }
          }
          frame "(ball) Calculate ROI" {
            n63 = local read "Number of Matches (Shape Detection 1)"() -> (w528:i32)
            n64 = Greater Than 0?(x=w528) -> (x > 0?=w529:bool)
            n65 = case shown="True" w529 {
              tunnel: [w530 w549] -> w526
              tunnel: w527 -> [w530 w549]
              frame False {
                w540 = 0 ("index")
                # "\"Black screen\", if no balls found"
                n66 = local read "ROI Descriptor COLOR Mask"() -> (w532:T3)
                n67 = local read "Ball index"() -> (w535:i32)
                n68 = Unbundle By Name(w532) -> ("Contours"=w533:T24)
                n69 = Index Array(array=w533, index=w535) -> (element=w538:T25)
                n70 = Unbundle By Name(w538) -> ("Coordinates"=w539:i32[])
                n71 = Replace Array Subset(array=w539, new element #1=w540, index #1=0 ("index"), new element #2=w540, index #2=1 ("index"), new element #3=w540, index #3=2 ("index"), new element #4=w540, index #4=3 ("index")) -> (w536:i32[])
                n72 = Bundle By Name(cluster=w538, "Coordinates"=w536) -> (w537:T25)
                n73 = Replace Array Subset(array=w533, new element=w537, index=w535) -> (w534:T24)
                n74 = Bundle By Name(cluster=w532, "Contours"=w534) -> (w531:T3)
                n75 = local write "ROI Descriptor COLOR Mask"(w531) -> ()
              }
              frame True {
                n76 = local read "ROI Descriptor COLOR Mask"() -> (w553:T3)
                n77 = local read "CircleRadius"() -> (w546:dbl)
                n78 = Divide(x=w546, y="divider (circle)") -> (x/y=w567:dbl)
                n79 = Unbundle By Name(w553) -> ("Contours"=w551:T24)
                n80 = local read "Ball index"() -> (w545:i32)
                n81 = local read "curX"() -> (w548:sgl)
                n82 = local read "curY"() -> (w547:sgl)
                n83 = Index Array(array=w551, index=w545) -> (element=w556:T25)
                n84 = Unbundle By Name(w556) -> ("Coordinates"=w561:i32[])
                n85 = Subtract(x=w548, y=w567) -> (x-y=w571:dbl)
                n86 = Subtract(x=w547, y=w567) -> (x-y=w570:dbl)
                n87 = Add(x=w548, y=w567) -> (x+y=w568:dbl)
                n88 = Add(x=w547, y=w567) -> (x+y=w569:dbl)
                n89 = To Long Integer(number=w571) -> (32bit integer=w560:i32)
                "x0 (circle)" <- w560
                n90 = To Long Integer(number=w570) -> (32bit integer=w559:i32)
                "y0 (circle)" <- w559
                n91 = To Long Integer(number=w568) -> (32bit integer=w558:i32)
                "x1 (circle)" <- w558
                n92 = To Long Integer(number=w569) -> (32bit integer=w557:i32)
                "y1 (circle)" <- w557
                n93 = Replace Array Subset(array=w561, new element #1=w560, index #1=0 ("index"), new element #2=w559, index #2=1 ("index"), new element #3=w558, index #3=2 ("index"), new element #4=w557, index #4=3 ("index")) -> (w554:i32[])
                n94 = Bundle By Name(cluster=w556, "Coordinates"=w554) -> (w555:T25)
                n95 = Replace Array Subset(array=w551, new element=w555, index=w545) -> (w550:T24)
                n96 = Bundle By Name(cluster=w553, "Contours"=w550) -> (w552:T3)
                n97 = local write "ROI Descriptor COLOR Mask"(w552) -> ()
              }
            }
          }
          frame "X align" {
            # "Align"
            # "Expansion State B"
            n98 = case shown="True" "Align X - t, Y - f" {
              tunnel: w574 -> [w578 w594]
              frame False {
                # "Bck"
                # "Fwd"
                # "Y align"
                n99 = local read "curY"() -> (w586:sgl)
                n100 = local read "Range"() -> (w581:dbl)
                n101 = Subtract(x="defY", y=w586) -> (x-y=w580:dbl)
                n102 = Multiply(x=w581, y=-1.0) -> (x*y=w579:dbl)
                n103 = Greater?(x=w580, y=w581) -> (0:w582:bool)
                n104 = Less?(x=w580, y=w579) -> (x < y?=w583:bool)
                n105 = Not Or(1:w583, 2:w582) -> (0:w584:bool)
                "Y is in range" <- w584
                n106 = case shown="True" w584 {
                  tunnel: w578 -> [_ w587]
                  frame False {
                  }
                  frame True {
                    n107 = local read "X is in range"() -> (w588:bool)
                    n108 = case shown="True" w588 {
                      tunnel: w587 -> [_ w590]
                      frame False {
                        n109 = local write "Align X - t, Y - f"(TRUE ("X - t, Y - f")) -> ()
                      }
                      frame True {
                        w591 = T21 [enum."Wait", enum."(image) get", enum."(myRIO) clean up", enum."(qsm) shutdown"] items=["(qsm) schedule", "(qsm) initialize", "(qsm) release", "(qsm) clean up", "(qsm) shutdown", "(myRIO) initialize", "(myRIO) clean up", "(myRIO) update ports", "(image) get", "(image) analyze", "(image) show", "(ball) Shape detection", "(ball) Calc ball indx", "(ball) Calculate ROI", "X align", "Wait", "Grab", "(pattern) Find Square", "(pattern) Calculate ROI", "(pattern) Analyze pattern", "(joystick) Joystick control", "Wait for button"] ("task")
                        n110 = call "enqueue_states.vi"("task"=w591, "queue in"=w590) -> ()  [unwired: 7 in, 2 out]
                      }
                    }
                  }
                }
                n111 = local write "Left-"(w583) -> ()
                n112 = local write "Left+"(w582) -> ()
                n113 = local write "Right+"(w582) -> ()
                n114 = local write "Right-"(w583) -> ()
              }
              frame True {
                # "X align"
                # "Right"
                # "Left"
                n115 = local read "curX"() -> (w595:sgl)
                n116 = Subtract(x="defX", y=w595) -> (x-y=w602:dbl)
                n117 = Multiply(x="Range", y=-1.0) -> (x*y=w601:dbl)
                n118 = Greater?(x=w602, y="Range") -> (0:w592:bool)
                n119 = Less?(x=w602, y=w601) -> (x < y?=w593:bool)
                n120 = Not(x=w593) -> (.not. x?=w598:bool)
                n121 = Not(x=w593) -> (.not. x?=w599:bool)
                n122 = And(x=w599, y=w598) -> (x .and. y?=w597:bool)
                "X is in range" <- w597
                n123 = case shown="True" w597 {
                  tunnel: w594 -> [_ w604]
                  frame False {
                  }
                  frame True {
                    n124 = local read "Y is in range"() -> (w605:bool)
                    n125 = case shown="True" w605 {
                      tunnel: w604 -> [_ w607]
                      frame False {
                        n126 = local write "Align X - t, Y - f"(FALSE ("X - t, Y - f")) -> ()
                      }
                      frame True {
                        w608 = T21 [enum."Wait", enum."(image) get", enum."(myRIO) clean up", enum."(qsm) shutdown"] items=["(qsm) schedule", "(qsm) initialize", "(qsm) release", "(qsm) clean up", "(qsm) shutdown", "(myRIO) initialize", "(myRIO) clean up", "(myRIO) update ports", "(image) get", "(image) analyze", "(image) show", "(ball) Shape detection", "(ball) Calc ball indx", "(ball) Calculate ROI", "X align", "Wait", "Grab", "(pattern) Find Square", "(pattern) Calculate ROI", "(pattern) Analyze pattern", "(joystick) Joystick control", "Wait for button"] ("task")
                        n127 = call "enqueue_states.vi"("task"=w608, "queue in"=w607) -> ()  [unwired: 7 in, 2 out]
                      }
                    }
                  }
                }
                n128 = local write "Left-"(w592) -> ()
                n129 = local write "Left+"(w593) -> ()
                n130 = local write "Right+"(w592) -> ()
                n131 = local write "Right-"(w593) -> ()
              }
            }
          }
          frame "Wait" {
            w619 = FALSE
            # "Expansion State D"
            n132 = local read "X is in range"() -> (w617:bool)
            n133 = local read "Y is in range"() -> (w616:bool)
            n134 = local write "Left-"(w619) -> ()
            n135 = local write "Left+"(w619) -> ()
            n136 = local write "Right+"(w619) -> ()
            n137 = local write "Right-"(w619) -> ()
            n138 = And(x=w617, y=w616) -> (x .and. y?=w618:bool)
            n139 = case shown="True" w618 {
              tunnel: w615 -> [w622 w627]
              tunnel: [w622 w627] -> w614
              tunnel: w613 -> [w621 w628]
              tunnel: [w621 w628] -> w612
              tunnel: w611 -> [w620 w623]
              tunnel: [w620 w626] -> w610
              tunnel: w609 -> [_ w624]
              frame False {
              }
              frame True {
                w625 = T21 [enum."(image) get", enum."(image) analyze", enum."(image) show", enum."(myRIO) update ports", enum."Grab", enum."Wait"] items=["(qsm) schedule", "(qsm) initialize", "(qsm) release", "(qsm) clean up", "(qsm) shutdown", "(myRIO) initialize", "(myRIO) clean up", "(myRIO) update ports", "(image) get", "(image) analyze", "(image) show", "(ball) Shape detection", "(ball) Calc ball indx", "(ball) Calculate ROI", "X align", "Wait", "Grab", "(pattern) Find Square", "(pattern) Calculate ROI", "(pattern) Analyze pattern", "(joystick) Joystick control", "Wait for button"] ("task")
                n140 = call "enqueue_states.vi"("task"=w625, "error in"=w623, "queue in"=w624) -> ("error out"=w626:errorcluster)  [unwired: 6 in, 1 out]
              }
            }
          }
          frame "Grab" {
            # "Expansion State E"
            n141 = flat-sequence {
              tunnel: w630 -> [w635]
              tunnel: [w634] -> w629
              frame #0 {
                n142 = xnode "M_PWM 2"("Duty Cycle"=0.5, "Frequency [Hz]"=400.0, "error in (no error)"=w635) -> ("error out"=w636:errorcluster)
                n143 = xnode "Digital output (1 sample) 3"("M+ (B/DIO5 (Pin 21))"="M+ (onGrab)", "error in (no error)"=w636) -> ("error out"=w634:errorcluster)
                n144 = Wait (ms)(milliseconds to wait="grab time (ms)") -> ()  [unwired: 1 out]
              }
            }
          }
          frame "(pattern) Find Square" {
            # "analyzed image buffer is\ncreated during the first\ncall of the Vision\nAssistant Express VI *only*\nwhen \"Create Destination\nImage\" option is enabled"
            # "Expansion State F"
            n145 = Unbundle By Name "Unbundle By Name"(w714) -> ("qsm.Webcam image ref"=w717:T2)
            n146 = call "Vision Assistant3"("Image In"=w717, "error in"=w710) -> ("Image Out"=w712:T2, "Calibrated Matches (Geometric Matching 1)"=→"Calibrated Matches (Geometric Matching 1)":T5[], "Number of Matches (Geometric Matching 1)"=→"Number of Matches (Geometric Matching 1)":i32, "error out"=w711:errorcluster)  [unwired: 22 in]
            n147 = Bundle By Name(cluster=w714, "qsm.Analyzed image ref"=w712) -> (w713:T1)
          }
          frame "(pattern) Calculate ROI" {
            # "Expansion State G"
            n148 = local read "Number of Matches (Geometric Matching 1)"() -> (w719:i32)
            n149 = Greater Than 0?(x=w719) -> (x > 0?=w724:bool)
            n150 = case shown="True" w724 {
              tunnel: [w726 w767] -> w722
              tunnel: w721 -> [w725 w766]
              frame False {
                w727 = 0 ("index")
                # "\"Black screen\", if no squares found"
                n151 = Unbundle By Name(w725) -> ("ROI Descriptor (Image Mask 1).Contours"=w734:T24)
                n152 = Index Array(array=w734, index=0) -> (element=w737:T25)
                n153 = Unbundle By Name(w737) -> ("Coordinates"=w736:i32[])
                n154 = Replace Array Subset(array=w736, new element #1=w727, index #1=0 ("index"), new element #2=w727, index #2=1 ("index"), new element #3=w727, index #3=2 ("index"), new element #4=w727, index #4=3 ("index")) -> (w738:i32[])
                n155 = Bundle By Name(cluster=w737, "Coordinates"=w738) -> (w739:T25)
                n156 = Replace Array Subset(array=w734, new element=w739, index=0) -> (w735:T24)
                n157 = Bundle By Name(cluster=w725, "ROI Descriptor (Image Mask 1).Contours"=w735) -> (w726:T1)
              }
              frame True {
                n158 = local read "Scale"() -> (w742:sgl)
                n159 = local read "Calibrated Matches (Geometric Matching 1)"() -> (w771:T5[])
                n160 = Index Array(array=w771, index=0) -> (element=w769:T5)
                n161 = Unbundle By Name(w769) -> ("Position"=w768:cluster{"x":sgl, "y":sgl}, "Scale"=→"Scale":sgl)
                n162 = Divide(x=w742, y="y") -> (x/y=w741:sgl)
                n163 = Unbundle(w768) -> ("x"=w761:sgl, "y"=w760:sgl)
                n164 = Unbundle By Name(w766) -> ("ROI Descriptor (Image Mask 1).Contours"=w764:T24)
                n165 = Index Array(array=w764, index=0) -> (element=w753:T25)
                n166 = Unbundle By Name(w753) -> ("Coordinates"=w755:i32[])
                n167 = Subtract(x=w761, y=w741) -> (x-y=w759:sgl)
                n168 = Subtract(x=w760, y=w741) -> (x-y=w758:sgl)
                n169 = Add(x=w761, y=w741) -> (x+y=w756:sgl)
                n170 = Add(x=w760, y=w741) -> (x+y=w757:sgl)
                n171 = To Long Integer(number=w759) -> (32bit integer=w750:i32)
                "x0" <- w750
                n172 = To Long Integer(number=w758) -> (32bit integer=w749:i32)
                "y0" <- w749
                n173 = To Long Integer(number=w756) -> (32bit integer=w748:i32)
                "x1" <- w748
                n174 = To Long Integer(number=w757) -> (32bit integer=w747:i32)
                "y1" <- w747
                n175 = Replace Array Subset(array=w755, new element #1=w750, index #1=0 ("index"), new element #2=w749, index #2=1 ("index"), new element #3=w748, index #3=2 ("index"), new element #4=w747, index #4=3 ("index")) -> (w752:i32[])
                n176 = Bundle By Name(cluster=w753, "Coordinates"=w752) -> (w751:T25)
                n177 = Replace Array Subset(array=w764, new element=w751, index=0) -> (w763:T24)
                n178 = Bundle By Name(cluster=w766, "ROI Descriptor (Image Mask 1).Contours"=w763) -> (w767:T1)
              }
            }
          }
          frame "(pattern) Analyze pattern" {
            n179 = Unbundle By Name(w779) -> ("qsm.Webcam image ref"=w781:T2, "ROI Descriptor (Image Mask 1)"=w777:T3)
            n180 = call "Vision Assistant4"("Image In"=w781, "ROI Descriptor (Image Mask 1)"=w777, "ROI Descriptor (Particle Classification 1)"=w777, "error in"=w772) -> ("Image Out"=w780:T2, "Class (Particle Classification 1)"=w775:string, "error out"=w773:errorcluster)  [unwired: 21 in]
            "Class (Particle Classification 1)" <- w775
            n181 = Decimal String To Number(string=w775) -> (number=w774:i32)  [unwired: 2 in, 1 out]
            n182 = Bundle By Name(cluster=w779, "qsm.Analyzed image ref"=w780, "Pattern class"=w774) -> (w778:T1)
          }
          frame "(joystick) Joystick control" {
            # "Cross (-1 - none; 0 - up; 90 - right; 180 - down; 270 - left)"
            n183 = shared-variable "My Computer\\KeyLibrary.lvlib\\Cross"() -> (w806:i32)  [unwired: 1 in, 1 out]
            n184 = shared-variable "My Computer\\KeyLibrary.lvlib\\A"() -> (w801:bool)  [unwired: 1 in, 1 out]
            n185 = shared-variable "My Computer\\KeyLibrary.lvlib\\B"() -> (w800:bool)  [unwired: 1 in, 1 out]
            n186 = shared-variable "My Computer\\KeyLibrary.lvlib\\X"() -> (w799:bool)  [unwired: 1 in, 1 out]
            n187 = shared-variable "My Computer\\KeyLibrary.lvlib\\Y"() -> (w790:bool)  [unwired: 1 in, 1 out]
            n188 = Equal?(x=w806, y=1) -> (x = y?=w794:bool)
            n189 = Equal?(x=w806, y=90) -> (x = y?=w793:bool)
            n190 = Equal?(x=w806, y=180) -> (x = y?=w792:bool)
            n191 = Equal?(x=w806, y=270) -> (x = y?=w791:bool)
            n192 = case shown="False" w790 {
              selector: w790 -> [w821 _]
              tunnel: w789 -> [w819 w857]
              tunnel: [w818 w857] -> w788
              frame False {
                n193 = Not(x=w821) -> (.not. x?=w820:bool)
                n194 = xnode "LED 3"("LED3"=w820, "error in (no error)"=w819) -> ("error out"=w818:errorcluster)
              }
              frame True {
              }
            }
            n195 = Or(x=w791, y=w799) -> (x .or. y?=w802:bool)
            n196 = local write "G-"(w802) -> ()
            n197 = Or(x=w794, y=w790) -> (x .or. y?=w805:bool)
            n198 = Or(x=w792, y=w801) -> (x .or. y?=w804:bool)
            n199 = local write "M+"(w805) -> ()
            n200 = local write "M-"(w804) -> ()
            n201 = Or(x=w793, y=w800) -> (x .or. y?=w803:bool)
            n202 = local write "G+"(w803) -> ()
            n203 = shared-variable "My Computer\\KeyLibrary.lvlib\\Forward"() -> (w785:bool)  [unwired: 1 in, 1 out]
            n204 = shared-variable "My Computer\\KeyLibrary.lvlib\\Left"() -> (w783:bool)  [unwired: 1 in, 1 out]
            n205 = shared-variable "My Computer\\KeyLibrary.lvlib\\Back"() -> (w784:bool)  [unwired: 1 in, 1 out]
            n206 = shared-variable "My Computer\\KeyLibrary.lvlib\\Right"() -> (w782:bool)  [unwired: 1 in, 1 out]
            n207 = Build Array(w785, w783, w784, w782) -> (w786:bool[])
            n208 = Or Array Elements(Boolean array=w786) -> (logical OR=w787:bool)
            n209 = case shown="True" w787 {
              selector: w787 -> [w809 _]
              tunnel: w785 -> [_ w817]
              tunnel: w784 -> [_ w816]
              tunnel: w783 -> [_ w811]
              tunnel: w782 -> [_ w810]
              frame False {
                n210 = local write "Right+"(w809) -> ()
                n211 = local write "Right-"(w809) -> ()
                n212 = local write "Left+"(w809) -> ()
                n213 = local write "Left-"(w809) -> ()
              }
              frame True {
                n214 = Or(x=w817, y=w810) -> (x .or. y?=w815:bool)
                n215 = Or(x=w816, y=w810) -> (x .or. y?=w812:bool)
                n216 = Or(x=w816, y=w811) -> (x .or. y?=w814:bool)
                n217 = Or(x=w811, y=w817) -> (x .or. y?=w813:bool)
                n218 = local write "Left+"(w815) -> ()
                n219 = local write "Left-"(w814) -> ()
                n220 = local write "Right+"(w813) -> ()
                n221 = local write "Right-"(w812) -> ()
              }
            }
          }
          frame "Wait for button" {
            n222 = while {
              stop <- w864 stop-if-true
              n223 = local read "Stop"() -> (w863:bool)
              n224 = Or(x="Look at ball", y=w863) -> (x .or. y?=w864:bool)
            }
            n225 = local write "Look at ball"(FALSE ("Look at ball")) -> ()
          }
        }
        n226 = Merge Errors(w51, w50) -> (w28:errorcluster)
        n227 = xnode "LED"("LED0"="x = y?", "error in (no error)"=w28) -> ("error out"=w27:errorcluster)
        n228 = Merge Errors(w19, w27) -> (w55:errorcluster)
        n229 = Unbundle By Name(w23) -> ("Pattern class"=w26:i32, "___Test___"=w18:i32[])
        "___Test___" <- w18
        n230 = local read "Number of Matches (Shape Detection 1)"() -> (w25:i32)
        n231 = local read "Ball index"() -> (w16:i32)
        n232 = Index Array(array=w18, index=w16) -> (element=w17:i32)
        n233 = Equal?(x=w26, y=w17) -> (x = y?=w20:bool)
        n234 = local write "x = y?"(w20) -> ()
        n235 = Greater Than 0?(x=w25) -> (x > 0?=w24:bool)
        n236 = case shown="False" w24 {
          tunnel: [w66 w72] -> w22
          tunnel: w23 -> [w65 w72]
          frame False {
            n237 = Unbundle By Name(w65) -> ("___Test___"=w62:i32[])
            n238 = for {
              N: 5 -> [w70]
              tunnel: [w71] -> w64
              tunnel: w62 -> [w68]
              n239 = Decrement(x=w70) -> (x-1=w69:i32)
              n240 = Replace Array Subset(array=w68, new element=20, index=w69) -> (w71:i32[])
            }
            n241 = Bundle By Name(cluster=w65, "___Test___"=w64) -> (w66:T1)
          }
          frame True {
          }
        }
      }
    }
    frame #1 {
      w868 = FALSE ("X is in range")
      n242 = local write "Align X - t, Y - f"(TRUE ("Align X - t, Y - f")) -> ()
      n243 = call <vilib>:"Simple Error Handler.vi"("error in (no error)"=w867) -> ("error out"=w866:errorcluster)  [unwired: 4 in, 4 out]
      "error out" <- w866
      n244 = local write "X is in range"(w868) -> ()
      n245 = local write "Y is in range"(w868) -> ()
      n246 = local write "Stop"(w868) -> ()
      n247 = local write "Look at ball"(w868) -> ()
      n248 = local write "x = y?"(w868) -> ()
      "data" <- w865
    }
  }
  n249 = call <vilib>:"Reset myRIO.vi"("error in (no error)"=w8) -> ()  [unwired: 10 in, 1 out]
